vi "Text control 2 v3.9.vi"() -> ()   [LabVIEW 2016]
panel:
  in  "Tab Control":enum32{"Main", "Other parameters"}(tab)
  out "Line running":i32
  out "Total lines":i32
  out "Path":path=path "C:/users/rlp38/09Apr2009LTtesting/test2.txt"
  out "I vs Vg":cluster{"Y data in":dbl[], "X data in":dbl[]}[](graph)
  out "Is":dbl format="%.2e"
  out "Id":dbl format="%.2e"
  out "Ig":dbl format="%.2e"
  out "Id max vs time":cluster{"Y data in":dbl[], "X data in":dbl[]}[](graph)
  out "Id min vs time":cluster{"Y data in":dbl[], "X data in":dbl[]}[](graph)
  out "I vs Vd":cluster{"Y data in":dbl[], "X data in":dbl[]}[](graph)
  in  "Program":string="#pulsedstressV d 0.03 20 0 0.5 0.0827 5\n#\n#itime s\n#gaterangemode l\n#drainrangemode l\n#serial /1Q #query pump\n#wait 1000 #wait 1 second\n#serial /1ZR #initialize pump\n#wait 20000 #wait 20 seconds\n#serial /1V300R #choose speed: 300 steps/s\n#wait 1000 #wait 1 second\n#serial /1O3R #go to port 3, counterclockwise rotation\n#wait 1000 #wait 1 second\n#serial /1A2400R #go to absolute position 2400\n#wait 1000 #wait 1 second\n#serial /1? #report absolute plunger position\n#serial /1V80R #set speed to 80 steps/s\n#serial /1O5 #switch to port 5, counterclockwise rotation\n#wait 200 #wait 200 milliseconds\n#serial /1A0R #go to absolute position 0 (= empty syringe)\n#serial /1? #report absolute plunger position\n#pulsed on 0.05 0 0.02\n#transfer d 1 -1 -0.1 -1 -1 0\n#wait-min 1\n#transfer d 1 -1 -0.1 -1 -1 0\n#output d 0 -1 -0.5 0 -1 -0.1\n#transfer d -10 40 1 5 40 35\n#transfer d -10 40 1 5 40 35\n#output d 0 40 20 0 40 1\n#\n#\n#sample 1 0.008 221 6 0.003\n#samplei 400e-6 200 6 0.002 0.1\n#vsu2pulse -10 4\n#\n#stressV 0.016 0.03 2e-4 0.1e-3 11\n#stressI 220e-7 0.08 15\n#transfer s -1 1 0.5 -0.005 0.005 0.005\n#output s 0 0 0 -0.008 0.008 0.002"
  out "Command running:":string="#output s 0 0 0 -0.008 0.008 0.002"
  out "Serial port output":string
  in  "Step delay /s":dbl format="%.2f"
  in  "Integration time (long)":dbl=0.32 min=0.04 max=2.0 step=0.02 format="%.2f"
  in  "Integration time (short)":dbl=0.0019 min=8e-05 max=0.0019 step=8e-05 format="%^.0e"
  in  "integration time":u32(slide) max=2 step=1 scale=0.0..2.0
  in  "delay time /s":dbl format="%.2f"
  in  "hold time /s":dbl format="%.2f"
  in  "Gate: Compliance":dbl=0.001 format="%.8f"
  in  "Drain: Compliance":dbl=0.001 format="%.8f"
  in  "Interrupt run":bool
  out "Elapsed Time":dbl caption="Elapsed Time (s)"
  in  "Units":u16(ring) items=["Seconds", "Minutes", "Hours"]
  in  "Time Offset":dbl caption="Set Start Time (s)"
  in  "Reset":bool
  in  "Auto Reset":bool
  in  "Gate Range\nmode":u16(ring) items=["Auto", "Limited", "Fixed"]
  in  "Gate Range":u8(slide)=6 max=11 scale=0.0..11.0
  in  "Source/Drain\nRange mode":u16(ring) items=["Auto", "Limited", "Fixed"]
  in  "Source/Drain Range":u8(slide)=6 max=11 scale=0.0..11.0
  in  "Panel Controls":T1={"Emergency Stop"=refnum, "TransGraph Max"=1e-05, "Text/Graph (text=false)"=TRUE} {"TransGraph Max" format="%.2e"}
  in  "Panel Controls 2":T2={"Emergency Stop"=refnum, "TransGraph Max"=1e-05, "Text/Graph (text=false)"=TRUE, "TransGraph Min"=1e-11} {"TransGraph Min" format="%.2e"; "TransGraph Max" format="%.2e"}
  in  "SMU4":cluster{"on/off":bool, "Voltage":dbl} {"Voltage" min=-100.0 max=100.0 format="%.2f"}
  in  "Full Reset":bool
  in  "Standby":T3
  in  "Delay before read (ms)":u32=1000
  in  "byte count":u32=64
  in  "Serial End Mode for Reads":u16(ring)=2 items=["None", "LastBit", "TermChar"]
  in  "Timeout (ms)":u32=10000
  in  "Enable Termination\nChar (T)":bool=TRUE
  in  "Termination char\n(0xA = '\\n' = LF)\n(0xD = '\\r' = CR)":u8=13 format="%.0x"
  in  "flow control":u16(ring) items=["None"=0, "XON/XOFF"=1, "RTS/CTS"=2, "DTR/DSR"=4]
  in  "stop bits":u16(ring)=10 items=["1.0"=10, "1.5"=15, "2.0"=20]
  in  "parity":u16(ring) items=["None", "Odd", "Even", "Mark", "Space"]
  in  "data bits":u16=8 min=5 max=8 step=1
  in  "VISA resource name":refnum<visa-resource-name>="COM6"
  in  "baud rate":u32=9600
  out "error out":errorcluster
  in  "Gate":T4={"Gate Start"=0.0, "Gate Stop"=2.0, "Gate Step (linear only)"=1.0, "Gate Compliance"=0.0001, "Gate PComp"=0.0, "Range mode"=0, "Range"=6} {"Range" max=11 scale=0.0..11.0; "Range mode" items=["Auto", "Limited", "Fixed"]; "Gate PComp" format="%^.2e"; "Gate Compliance" format="%^.2e"; "Gate Step (linear only)" format="%^.4e"; "Gate Stop" format="%^.4e"; "Gate Start" format="%^.4e"}
  in  "Drain 2":T5={"Drain Start"=0.0, "Drain Stop"=2.0, "Drain Compliance"=0.0001, "Drain Step"=1.0, "Drain PComp"=0.0, "Range mode"=0, "Range"=6} {"Range" max=11 scale=0.0..11.0; "Range mode" items=["Auto", "Limited", "Fixed"]; "Drain PComp" format="%^.2e"; "Drain Step" format="%^.4e"; "Drain Compliance" format="%^.2e"; "Drain Stop" format="%^.4e"; "Drain Start" format="%^.4e"}
  in  "Timings 2":T6={"integration time"=0, "Short/Long integration time"=0.00064, "hold time (sec)"=0.0, "delay time (sec)"=0.0, "Step Time (0 disables)"=0.0, "sweep method"=0, "Pulse period"=0.005, "Base voltage"=0.0, "Pulse width"=0.0005} {"Pulse width" min=0.0005 max=0.1 step=0.0001 format="%.4f"; "Base voltage" format="%^.4e"; "Pulse period" min=0.005 max=1.0 step=0.0001 format="%.4f"; "sweep method" items=["Continuous", "Pulsed"]; "Step Time (0 disables)" format="%.2f"; "delay time (sec)" format="%.4f"; "hold time (sec)" format="%.4f"; "Short/Long integration time" format="%^.0e"; "integration time" scale=0.0..2.0}
  # "Time"
  # "1\n2\n3\n4\n5\n6\n7\n8\n9\n10\n11\n12\n13\n14\n15\n16\n17\n18\n19\n20\n21\n22\n23\n24\n25"
  # "Syntax:\nitime [s|m|l]\ngaterangemode [a|l|f]\ndrainrangemode [a|l|f]\npulsed [on|off] PulsePeriod(sec) PulseBaseVoltage PulseONWidth(sec)\nstandby [on l off]\nwait NumMilliseconds\nwait-min NumMinutes\n# texthere = comment\ntransfer [s|d] VgStart VgStop VgStep VdStart VdStop VdStep\noutput [s|d] VgStart VgStop VgStep VdStart VdStop VdStep\nsample Vg Vd NumSamples Time(s) SampleInterval(s)\nsamplei Idg NumSamples Time(s) SampleInterval(s) VDGcompliance\n100 samples is approximately 13 seconds with medium integration\n# if in doubt use SampleInterval(s) = 0.004\nstressV VG VD IGcompliance IDcompliance Duration(sec)\nstressI IDG VDGcompliance Duration(sec)\nvsu2pulse Bias Duration(s)\npulsedstressV [s|d] VEstop VgON VgOFF Period(s) PulseONwidth(s) Vd\nsample-fpp Vg Vd NumSamples Time\nresample-fpp Vg Vd\ntransfer-fpp [s|d] VgStart VgStop VgStep VdStart VdStop VdStep\noutput-fpp [s|d] VgStart VgStop VgStep VdStart VdStop VdStep\nserial SerialPortCommand"
  # "Serial port settings"
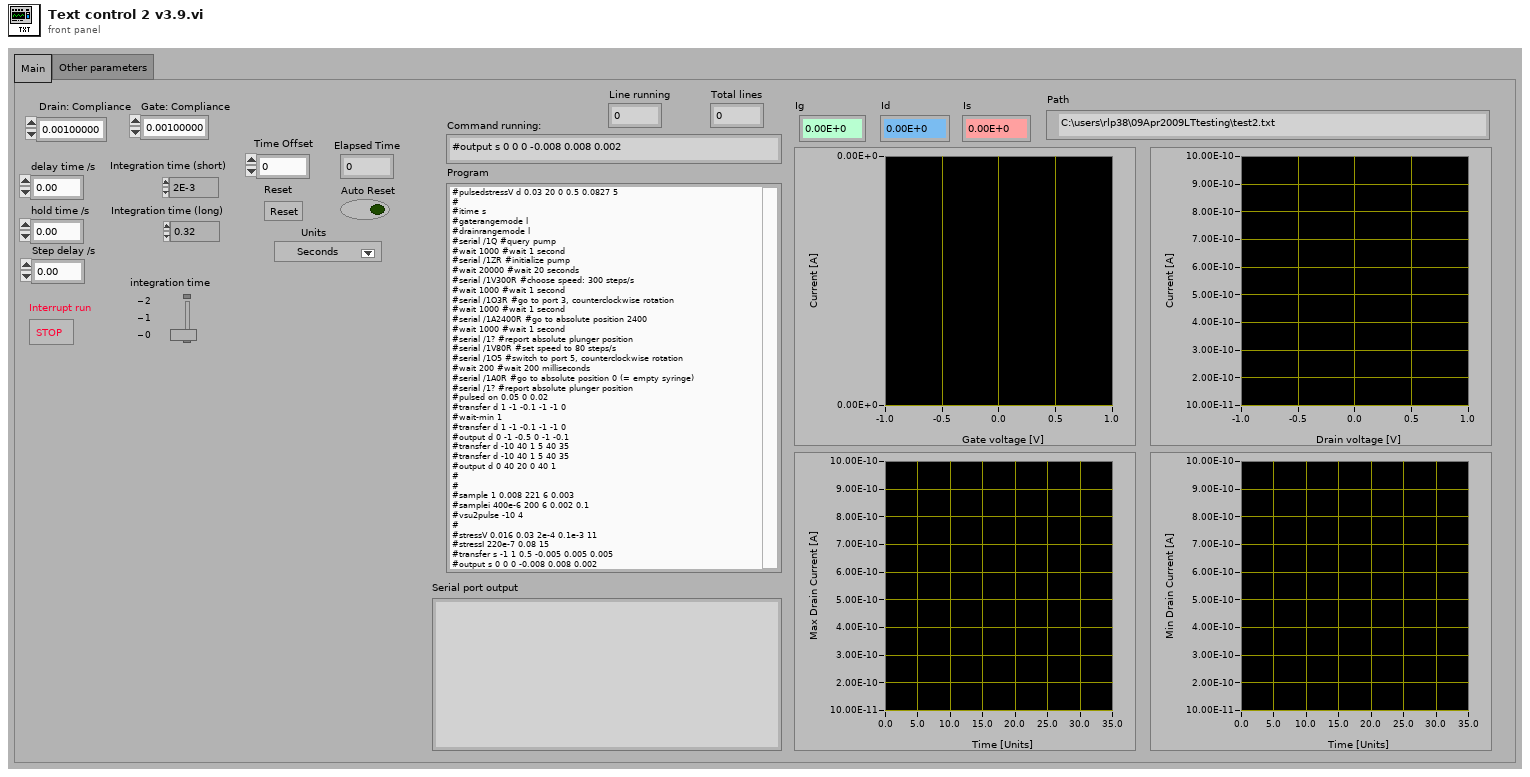
[diagram p1: front panel]
types:
  T1 = cluster{"Emergency Stop":refnum<vi>, "TransGraph Max":dbl, "Text/Graph (text=false)":bool}
  T2 = cluster{"Emergency Stop":refnum<vi>, "TransGraph Max":dbl, "Text/Graph (text=false)":bool, "TransGraph Min":dbl}
  T3 = cluster{"Gate Standby":bool, "Drain Standby":bool}
  T4 = cluster{"Gate Start":dbl, "Gate Stop":dbl, "Gate Step (linear only)":dbl, "Gate Compliance":dbl, "Gate PComp":dbl, "Range mode":u16, "Range":u8}
  T5 = cluster{"Drain Start":dbl, "Drain Stop":dbl, "Drain Compliance":dbl, "Drain Step":dbl, "Drain PComp":dbl, "Range mode":u16, "Range":u8}
  T6 = cluster{"integration time":u32, "Short/Long integration time":dbl, "hold time (sec)":dbl, "delay time (sec)":dbl, "Step Time (0 disables)":dbl, "sweep method":u16, "Pulse period":dbl, "Base voltage":dbl, "Pulse width":dbl}
  T7 = enum16{"open", "replace", "create", "open or create", "replace or create", "replace or create with confirmation"}
  T8 = cluster{"V2 Start":dbl, "V2 Step":dbl, "Number of points":i32}
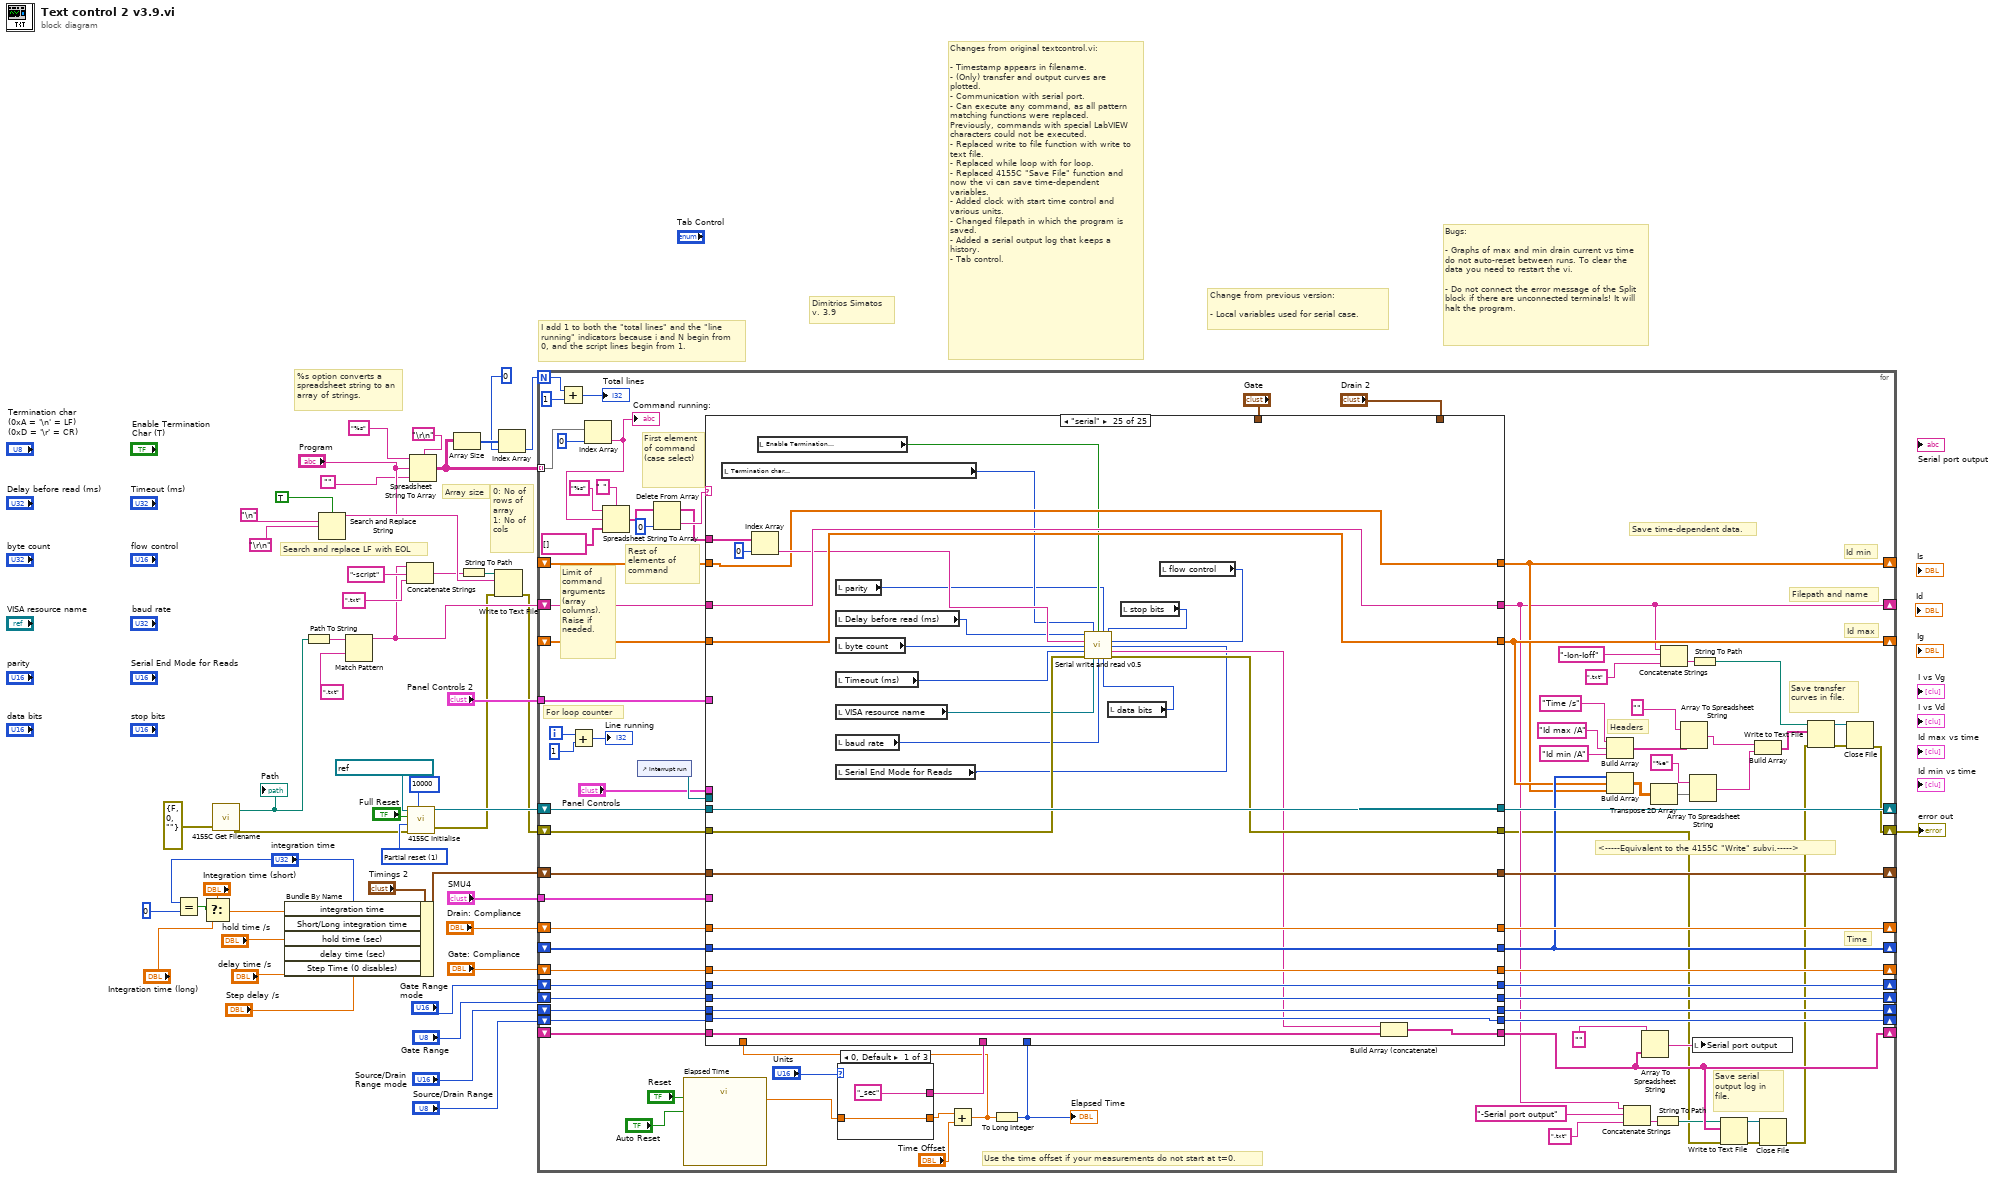
[diagram p0: block diagram]
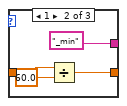
[diagram p2: hidden frame]
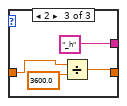
[diagram p3: hidden frame]
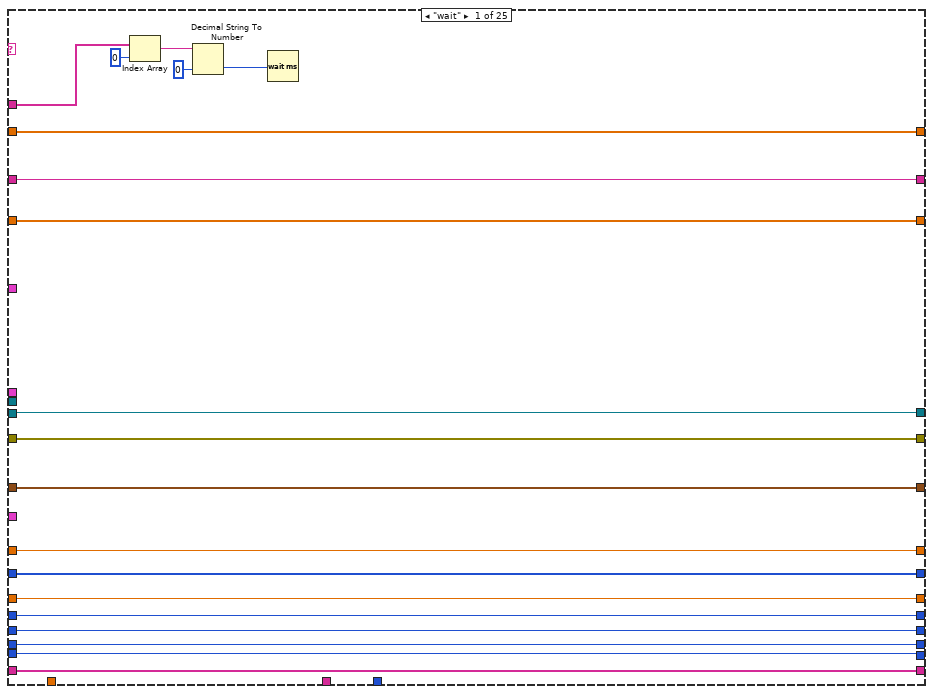
[diagram p4: hidden frame]
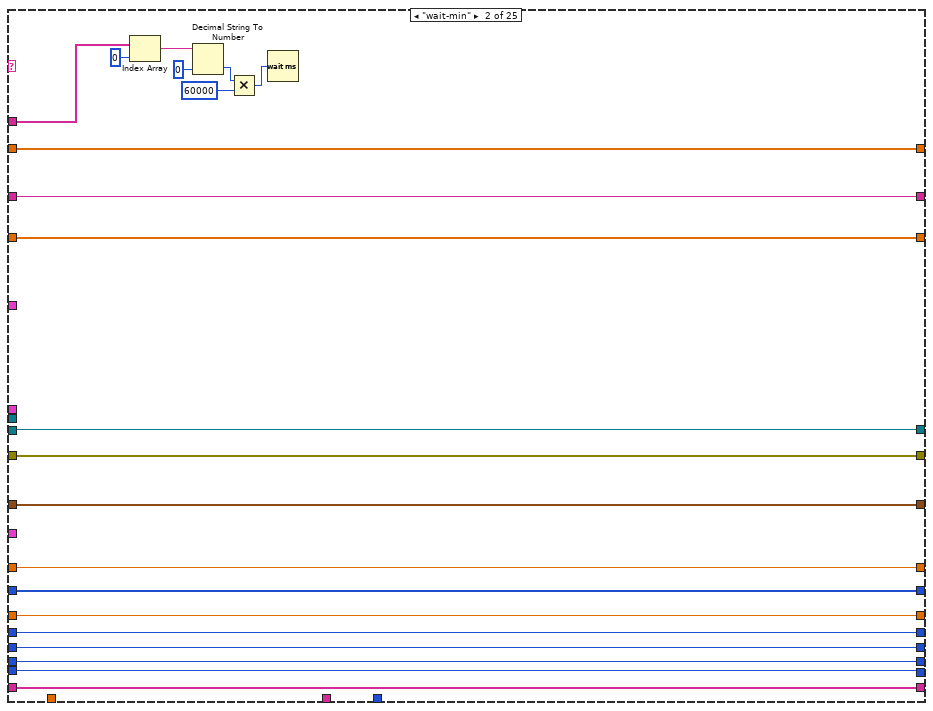
[diagram p5: hidden frame]
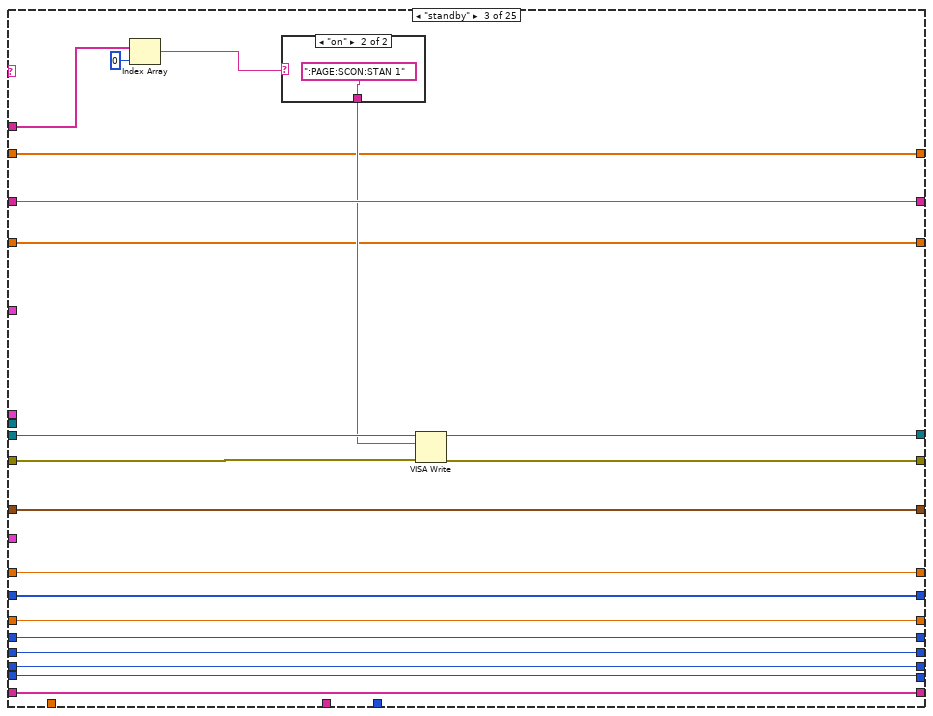
[diagram p6: hidden frame]
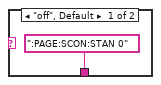
[diagram p7: hidden frame]
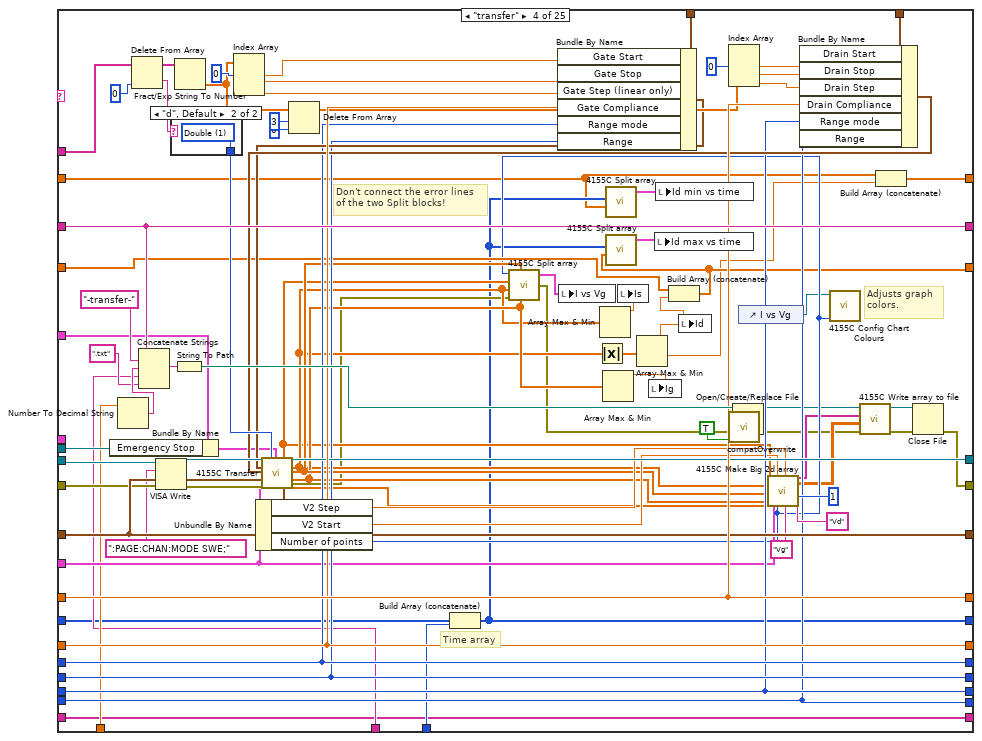
[diagram p8: hidden frame]
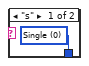
[diagram p9: hidden frame]
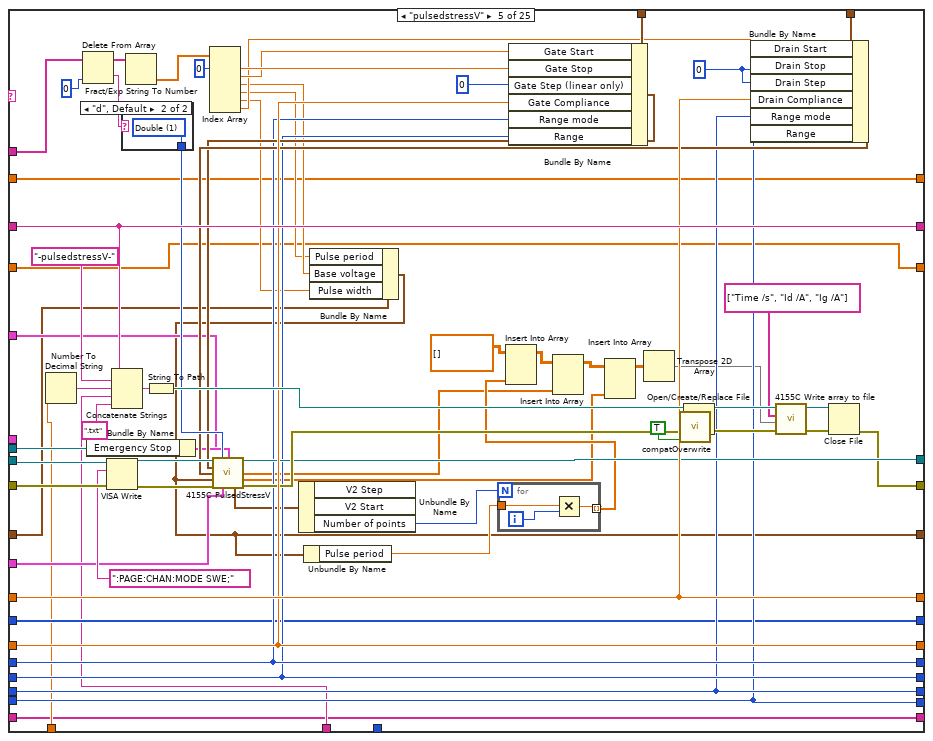
[diagram p10: hidden frame]
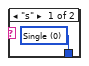
[diagram p11: hidden frame]
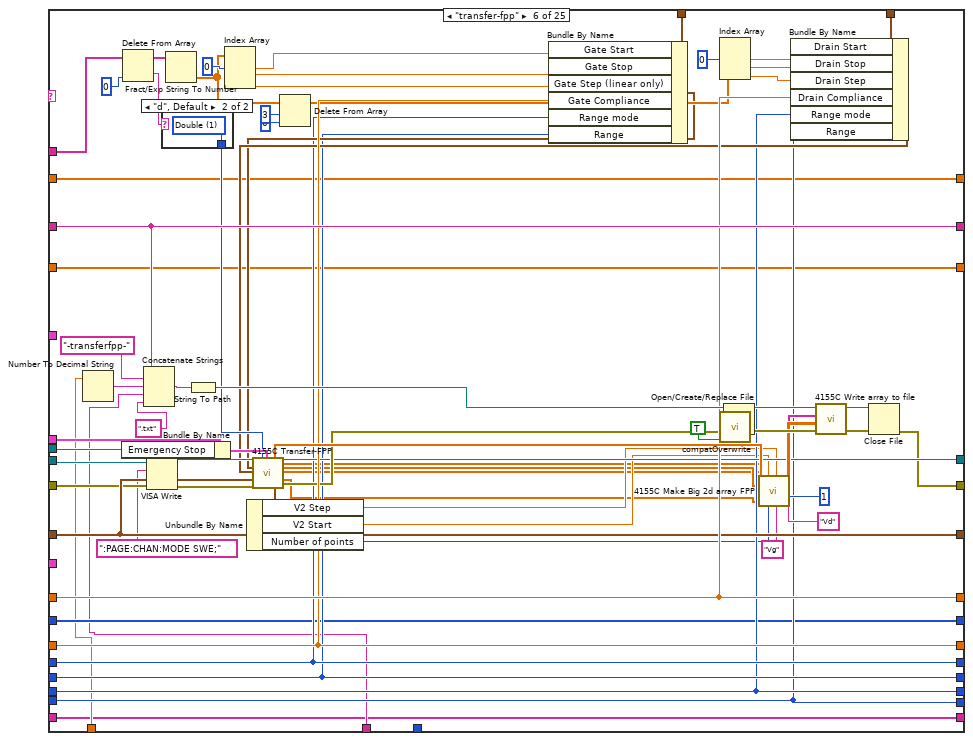
[diagram p12: hidden frame]
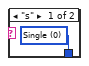
[diagram p13: hidden frame]
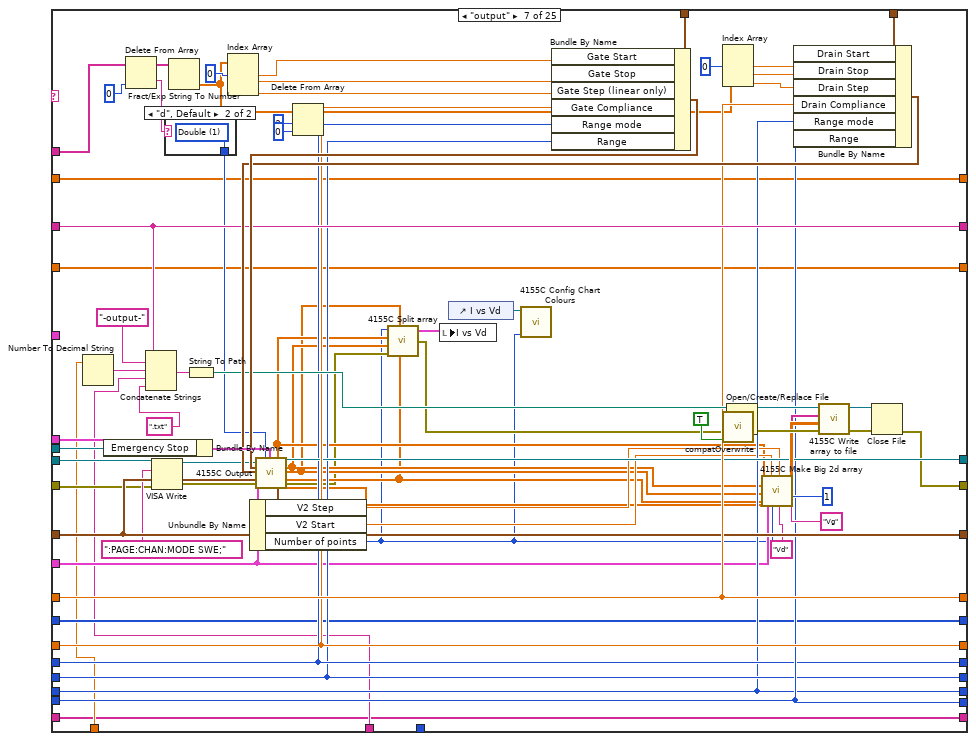
[diagram p14: hidden frame]
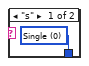
[diagram p15: hidden frame]
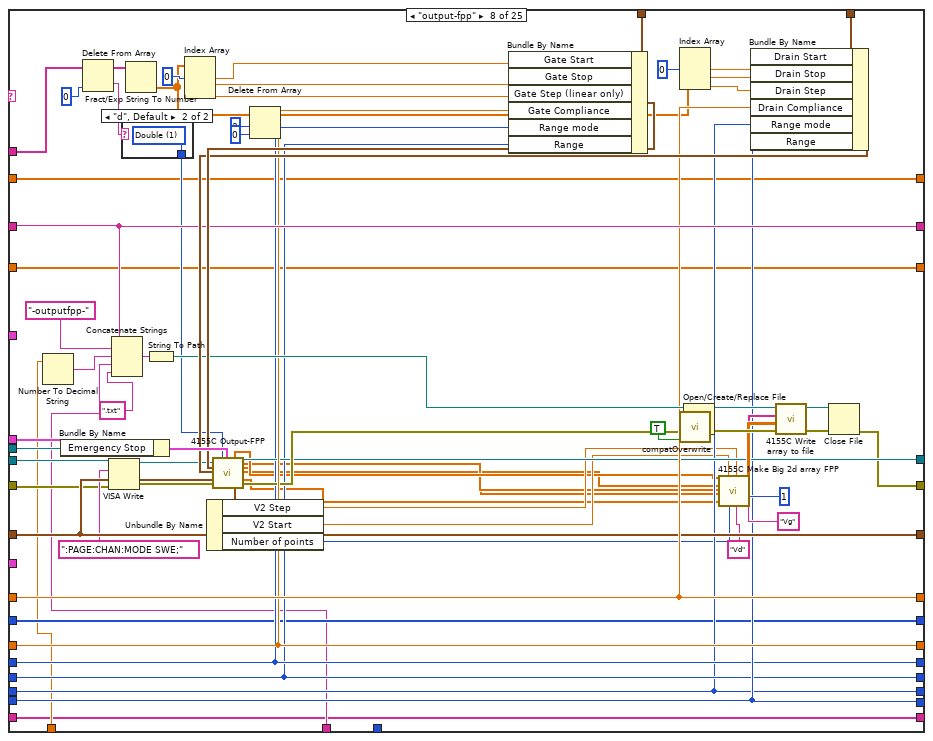
[diagram p16: hidden frame]
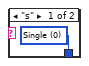
[diagram p17: hidden frame]
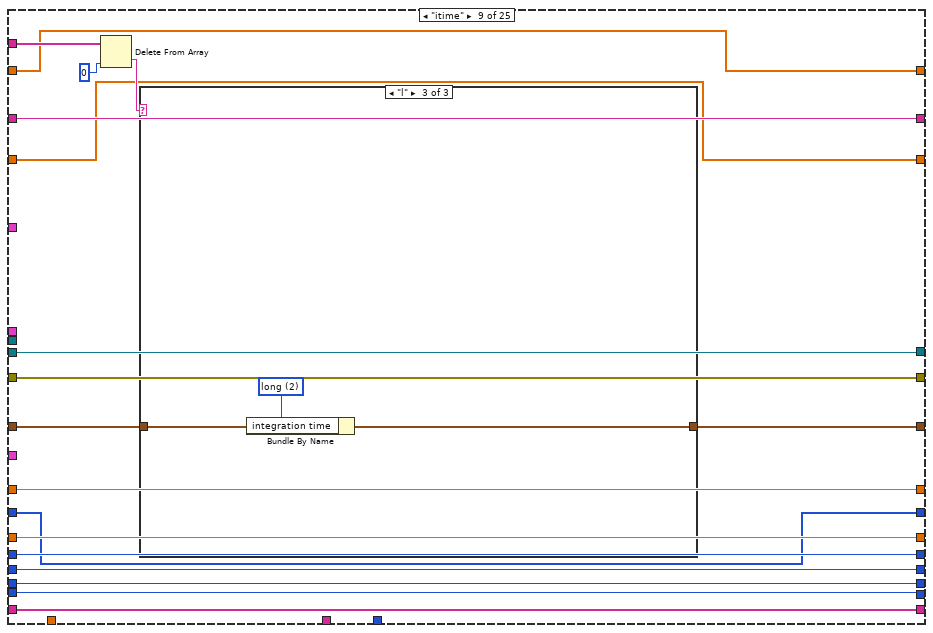
[diagram p18: hidden frame]
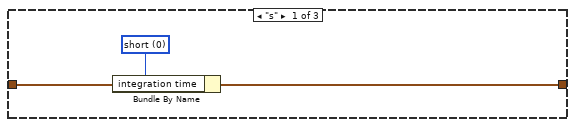
[diagram p19: hidden frame]
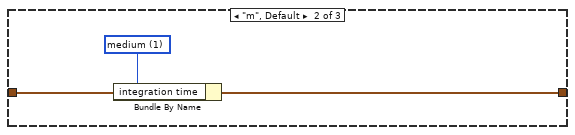
[diagram p20: hidden frame]
diagram:
  w40 = u16 1 items=["Reset All", "Partial reset"] ("Type of reset")
  # "Change from previous version:\n\n- Local variables used for serial case."
  # "I add 1 to both the \"total lines\" and the \"line running\" indicators because i and N begin from 0, and the script lines begin from 1."
  # "Bugs:\n\n- Graphs of max and min drain current vs time do not auto-reset between runs. To clear the data you need to restart the vi.\n\n- Do not connect the error message of the Split block if there are unconnected terminals! It will halt the program."
  # "Array size"
  # "%s option converts a spreadsheet string to an array of strings."
  # "0: No of rows of array\n1: No of cols"
  # "Dimitrios Simatos\nv. 3.9"
  # "Changes from original textcontrol.vi:\n\n- Timestamp appears in filename.\n- (Only) transfer and output curves are plotted.\n- Communication with serial port.\n- Can execute any command, as all pattern matching functions were replaced. Previously, commands with special LabVIEW characters could not be executed.\n- Replaced write to file function with write to text file.\n- Replaced while loop with for loop.\n- Replaced 4155C \"Save File\" function and now the vi can save time-dependent variables.\n- Added clock with start time control and various units.\n- Changed filepath in which the program is saved.\n- Added a serial output log that keeps a history.\n- Tab control."
  # "Search and replace LF with EOL"
  n1 = Equal?(x="integration time", y=u32 0) -> (x = y?=w44:bool)
  n2 = Select(t="Integration time (short)", s=w44, f="Integration time (long)") -> (s? t:f=w48:dbl)
  n3 = call "4155C Get Filename.vi"("error in (no error)"=errorcluster {"status"=FALSE, "code"=0, "source"=""}) -> ("error out"=w35:errorcluster, "path"=w10:path)  [unwired: 2 in, 1 out]
  "Path" <- w10
  n4 = Bundle By Name(cluster="Timings 2", "integration time"="integration time", "Short/Long integration time"=w48, "hold time (sec)"="hold time /s", "delay time (sec)"="delay time /s", "Step Time (0 disables)"="Step delay /s") -> (w33:T6)
  n5 = Path To String(path=w10) -> (string=w11:string)
  n6 = Search and Replace String(replace all?=TRUE ("replace all? (F)"), input string="Program", search string="\n", replace string="\r\n") -> (result string=w23:string)  [unwired: 4 in, 3 out]
  n7 = Match Pattern(string=w11, regular expression=".txt") -> (before substring=w5:string)  [unwired: 1 in, 3 out]
  n8 = Concatenate Strings(w5, "-script" ("Prefix"), ".txt" ("regular expression")) -> (w4:string)
  n9 = call "4155C Initialise.vi"("VISA resource name in"=refnum<visa-resource-name> "GPIB0::14::INSTR", "Reset"="Full Reset", "Type of reset"=w40, "error in (no error)"=w35, "VISA Timeout Value"=u32 10000) -> ("VISA Resource Name out"=w34:refnum<visa-resource-name>, "error out"=w2:errorcluster)
  n10 = Spreadsheet String To Array(delimiter (Tab)="\r\n", format string="%s", spreadsheet string="Program", array type (2D Dbl)="") -> (array=w14:string[][])
  n11 = Array Size(array=w14) -> (size(s)=w18:i32[])
  n12 = String To Path(string=w4) -> (path=w3:path)
  n13 = Write to Text File(file (use dialog)=w3, text=w23, error in=w2) -> (error out=w1:errorcluster)  [unwired: 1 in, 2 out]
  n14 = Index Array(array=w18, index=0) -> (element=w16:i32)
  n15 = for {
    N: w16 -> [w68]
    tunnel: "SMU4" -> [w113]
    shift-left: "Source/Drain Range" -> [w118]
    shift-right: [w114] -> _
    shift-left: "Source/Drain\nRange mode" -> [w119]
    shift-right: [w115] -> _
    shift-left: "Gate Range" -> [w120]
    shift-right: [w116] -> _
    shift-left: "Gate Range\nmode" -> [w121]
    shift-right: [w117] -> _
    shift-left: "Gate: Compliance" -> [w130]
    shift-right: [w126] -> _
    shift-left: "Drain: Compliance" -> [w131]
    shift-right: [w127] -> _
    shift-left: w33 -> [w132]
    shift-right: [w128] -> _
    shift-left: w1 -> [w133]
    shift-right: [w76] -> w9
    shift-left: w34 -> [w134]
    shift-right: [w129] -> _
    shift-left: w5 -> [w135]
    shift-right: [w52] -> _
    tunnel: "Panel Controls 2" -> [w112]
    shift-right: [w80] -> _
    shift-left: _ -> [w111]
    shift-right: [w81] -> _
    shift-left: _ -> [w107]
    tunnel: w14 -> [w105] mode=indexing
    shift-right: [w74] -> _
    shift-left: _ -> [w75]
    shift-right: [w57] -> _
    shift-left: _ -> [w60]
    i -> [w63]
    # "Save serial output log in file."
    # "For loop counter"
    # "<-----Equivalent to the 4155C \"Write\" subvi.----->"
    # "Headers"
    # "Save transfer curves in file."
    # "Filepath and name"
    # "Save time-dependent data."
    # "Use the time offset if your measurements do not start at t=0."
    # "Time"
    # "Rest of elements of command"
    # "Id min"
    # "Id max"
    # "Limit of command arguments (array columns). Raise if needed."
    # "First element of command\n(case select)"
    n16 = Add(x=w68, y=1) -> (x+y=→"Total lines":i32)
    n17 = Add(x=w63, y=1) -> (x+y=→"Line running":i32)
    n18 = Index Array(array=w105, index=0 ("line index")) -> (element=w100:string)
    "Command running:" <- w100
    n19 = Spreadsheet String To Array(delimiter (Tab)=" ", format string="%s", spreadsheet string=w100, array type (2D Dbl)=string[] []) -> (array=w97:string[])
    n20 = control-ref of="Interrupt run"() -> (w125:refnum<vi>)
    n21 = Delete From Array(array=w97, index=0) -> (deleted portion=w98:string, array with subset deleted=w96:string[])  [unwired: 1 in]
    n22 = call "Elapsed Time"("Reset"="Reset", "Auto Reset"="Auto Reset") -> ("Elapsed Time (s)"=w108:dbl)  [unwired: 10 in, 7 out]
    n23 = case shown="0, Default" "Units" {
      tunnel: ["_sec" "_min" "_h"] -> w109
      tunnel: [w136 w140 w143] -> w70
      tunnel: w108 -> [w136 w139 w144]
      frame 0, Default {
      }
      frame 1 {
        n24 = Divide(x=w139, y=60.0) -> (x/y=w140:dbl)
      }
      frame 2 {
        n25 = Divide(x=w144, y=3600.0) -> (x/y=w143:dbl)
      }
    }
    n26 = Add(x=w70, y="Time Offset") -> (x+y=w69:dbl)
    n27 = To Long Integer(number=w69) -> (32bit integer=w106:i32)
    "Elapsed Time" <- w106
    n28 = case shown="\"serial\"" w98 {
      tunnel: w96 -> [w164 w185 w205 w282 w348 w419 w496 w568 w608 w636 w665 w692 w715 w731 _ _ w841 w904 _ w973 w1019 w1063 w1135 w1199 w1221]
      tunnel: w135 -> [w159 w181 w203 w289 w355 w427 w503 w576 w597 w625 w657 w685 w709 w724 w745 w789 w819 w886 w919 w960 w1006 w1051 w1129 w1195 w1223]
      tunnel: w134 -> [w158 w180 w194 w260 w339 w396 w472 w544 w598 w626 w658 w686 w710 w725 w750 w791 w847 w910 w923 w979 w1025 w1069 w1141 w1153 w1227]
      tunnel: w133 -> [w157 w179 w193 w259 w338 w395 w469 w541 w599 w627 w659 w687 w711 w726 w749 w762 w846 w909 w922 w978 w1024 w1068 w1140 w1152 w1226]
      tunnel: w132 -> [w156 w178 w202 w285 w314 w423 w499 w572 w607 w635 w656 w684 w708 w723 w748 w786 w810 w878 w928 w953 w999 w1044 w1128 w1194 w1228]
      tunnel: w131 -> [w155 w177 w201 w287 w353 w425 w501 w574 w606 w634 w664 w691 w714 w730 w747 w771 w845 w908 w931 w977 w1023 w1067 w1139 w1203 w1229]
      tunnel: w130 -> [w154 w176 w200 w286 w352 w424 w500 w573 w605 w633 w663 w690 w713 w729 w746 w772 w820 w887 w930 w961 w1007 w1052 w1130 w1196 w1231]
      tunnel: [w158 w180 w192 w284 w350 w421 w498 w570 w598 w626 w658 w686 w710 w725 w750 w791 w811 w860 w921 w954 w1000 w1045 w1081 w1155 w1227] -> w129
      tunnel: [w157 w179 w191 w283 w349 w420 w497 w569 w599 w627 w659 w687 w711 w726 w749 w761 w821 w861 w920 w962 w1008 w1053 w1080 w1154 w1225] -> w51
      tunnel: [w156 w178 w202 w285 w310 w423 w499 w572 w600 w628 w656 w684 w708 w723 w748 w786 w810 w878 w928 w953 w999 w1044 w1128 w1194 w1228] -> w128
      tunnel: [w155 w177 w201 w287 w353 w425 w501 w574 w606 w634 w664 w691 w714 w730 w747 w771 w845 w908 w931 w977 w1023 w1067 w1139 w1203 w1229] -> w127
      tunnel: [w154 w176 w200 w286 w352 w424 w500 w573 w605 w633 w663 w690 w713 w729 w746 w772 w820 w887 w930 w961 w1007 w1052 w1130 w1196 w1231] -> w126
      tunnel: [w159 w181 w203 w289 w355 w427 w503 w576 w597 w625 w657 w685 w709 w724 w745 w789 w819 w886 w919 w960 w1006 w1051 w1129 w1195 w1223] -> w52
      tunnel: w125 -> [_ _ _ w292 w359 w432 w507 w580 _ _ _ _ _ _ _ _ w816 w883 _ w959 w1005 w1050 w1101 w1171 _]
      tunnel: "Gate" -> [_ _ _ w269 w342 w406 w483 w555 _ _ _ _ _ _ _ _ _ _ _ _ _ _ _ _ _]
      tunnel: "Drain 2" -> [_ _ _ w268 w341 w405 w482 w554 _ _ _ _ _ _ _ _ _ _ _ _ _ _ _ _ _]
      tunnel: "Panel Controls" -> [_ _ _ _ _ w404 w481 w553 _ _ _ _ _ _ _ _ _ _ _ _ _ _ _ _ _]
      tunnel: w121 -> [w153 w175 w199 w253 w332 w389 w467 w539 w604 w632 _ w683 w707 w722 w744 w773 w806 w874 w924 w949 w995 w1040 w1124 w1190 w1232]
      tunnel: w120 -> [w152 w174 w198 w252 w331 w388 w466 w538 w603 w631 w662 _ w698 w728 w743 w774 w807 w875 w925 w950 w996 w1041 w1125 w1191 w1233]
      tunnel: w119 -> [w151 w173 w197 w251 w330 w387 w465 w537 w602 w630 w661 w689 w712 _ w742 w775 w808 w876 w926 w951 w997 w1042 w1126 w1192 w1234]
      tunnel: w118 -> [w150 w172 w196 w250 w329 w386 w468 w540 w601 w629 w660 w688 _ w727 w741 w776 w809 w877 w927 w952 w998 w1043 w1127 w1193 w1235]
      tunnel: [w153 w175 w199 w253 w332 w389 w467 w539 w604 w632 w655 w683 w707 w722 w744 w773 w806 w874 w924 w949 w995 w1040 w1124 w1190 w1232] -> w117
      tunnel: [w152 w174 w198 w252 w331 w388 w466 w538 w603 w631 w662 w675 w698 w728 w743 w774 w807 w875 w925 w950 w996 w1041 w1125 w1191 w1233] -> w116
      tunnel: [w151 w173 w197 w251 w330 w387 w465 w537 w602 w630 w661 w689 w712 w721 w742 w775 w808 w876 w926 w951 w997 w1042 w1126 w1192 w1234] -> w115
      tunnel: [w150 w172 w196 w250 w329 w386 w468 w540 w601 w629 w660 w688 w699 w727 w741 w776 w809 w877 w927 w952 w998 w1043 w1127 w1193 w1235] -> w114
      tunnel: w113 -> [_ _ _ w245 w326 _ w461 _ _ _ _ _ _ _ _ _ _ _ _ _ _ _ _ _ _]
      tunnel: w112 -> [_ _ _ w243 w325 _ _ _ _ _ _ _ _ _ _ _ _ _ _ _ _ _ _ _ _]
      tunnel: [w149 w168 w189 w220 w302 w376 w458 w526 w596 w623 w654 w674 w697 w720 w740 w757 w798 w858 w918 w938 w988 w1034 w1078 w1148 w1224] -> w80
      tunnel: w111 -> [w149 w168 w189 w234 w302 w376 w458 w526 w596 w623 w654 w674 w697 w720 w740 w757 w798 w858 w918 w938 w988 w1034 w1078 w1148 w1224]
      tunnel: w69 -> [_ _ _ w230 w299 w374 w455 w523 _ _ _ _ _ _ _ w755 w796 w855 _ w935 w985 w1031 w1075 w1144 _]
      tunnel: w109 -> [_ _ _ w227 w298 w372 w454 w522 _ _ _ _ _ _ _ w753 w794 w854 _ w934 w984 w1030 w1074 w1145 _]
      tunnel: w106 -> [_ _ _ w221 _ _ _ _ _ _ _ _ _ _ _ _ _ _ _ _ _ _ _ _ _]
      tunnel: [w148 w167 w188 w218 w301 w375 w457 w525 w595 w622 w653 w673 w696 w719 w739 w756 w797 w857 w917 w937 w987 w1033 w1077 w1147 w1230] -> w81
      tunnel: w107 -> [w148 w167 w188 w226 w301 w375 w457 w525 w595 w622 w653 w673 w696 w719 w739 w756 w797 w857 w917 w937 w987 w1033 w1077 w1147 w1230]
      tunnel: [w147 w166 w187 w216 w297 w371 w453 w521 w594 w621 w652 w672 w695 w718 w738 w752 w793 w853 w916 w933 w983 w1029 w1073 w1143 w1219] -> w74
      tunnel: w75 -> [w147 w166 w187 w215 w297 w371 w453 w521 w594 w621 w652 w672 w695 w718 w738 w752 w793 w853 w916 w933 w983 w1029 w1073 w1143 w1219]
      tunnel: [w146 w165 w186 w208 w296 w370 w443 w520 w593 w620 w651 w671 w694 w717 w737 w751 w792 w852 w915 w932 w982 w1028 w1072 w1142 w1217] -> w57
      tunnel: w60 -> [w146 w165 w186 w208 w296 w370 w443 w520 w593 w620 w651 w671 w694 w717 w737 w751 w792 w852 w915 w932 w982 w1028 w1072 w1142 w1216]
      frame "wait" {
        n29 = Index Array(array=w164, index=0 ("Index")) -> (element=w162:string)
        n30 = Decimal String To Number(string=w162, default (0L)=u32 0) -> (number=w161:u32)  [unwired: 1 in, 1 out]
        n31 = Wait (ms)(milliseconds to wait=w161) -> ()  [unwired: 1 out]
      }
      frame "wait-min" {
        n32 = Index Array(array=w185, index=0 ("Index")) -> (element=w183:string)
        n33 = Decimal String To Number(string=w183, default (0L)=u32 0) -> (number=w171:u32)  [unwired: 1 in, 1 out]
        n34 = Multiply(x=w171, y=u32 60000) -> (x*y=w170:u32)
        n35 = Wait (ms)(milliseconds to wait=w170) -> ()  [unwired: 1 out]
      }
      frame "standby" {
        n36 = Index Array(array=w205, index=0 ("Index")) -> (element=w195:string)
        n37 = case shown="\"on\"" w195 {
          tunnel: [":PAGE:SCON:STAN 0" ":PAGE:SCON:STAN 1"] -> w190
          frame "off", Default {
          }
          frame "on" {
          }
        }
        n38 = VISA Write(VISA resource name=w194, write buffer=w190, error in (no error)=w193) -> (VISA resource name out=w192:refnum<visa-resource-name>, error out=w191:errorcluster)  [unwired: 1 out]
      }
      frame "transfer" {
        # "Don't connect the error lines\nof the two Split blocks!"
        # "Adjusts graph colors."
        # "Time array"
        n39 = Bundle By Name(cluster=w243, "Emergency Stop"=w292) -> (w244:T2)
        n40 = Number To Decimal String(number=w230) -> (decimal integer string=w229:string)  [unwired: 1 in]
        n41 = Delete From Array(array=w282, index=0 ("Index")) -> (deleted portion=w280:string, array with subset deleted=w279:string[])  [unwired: 1 in]
        n42 = Concatenate Strings(w289, "-transfer-" ("Prefix"), w229, w227, ".txt" ("Suffix")) -> (w291:string)
        n43 = VISA Write(VISA resource name=w260, write buffer=":PAGE:CHAN:MODE SWE;" ("write buffer (\"\")"), error in (no error)=w259) -> (VISA resource name out=w257:refnum<visa-resource-name>, error out=w258:errorcluster)  [unwired: 1 out]
        n44 = case shown="\"d\", Default" w280 {
          tunnel: [w294 w295] -> w278
          frame "s" {
            w294 = u16 0 items=["Single", "Double"] ("sweep mode")
          }
          frame "d", Default {
            w295 = u16 1 items=["Single", "Double"] ("sweep mode")
          }
        }
        n45 = String To Path(string=w291) -> (path=w288:path)
        n46 = Fract/Exp String To Number(string=w279) -> (number=w264:dbl[])  [unwired: 3 in, 1 out]
        n47 = Index Array(array=w264, index #1=0 ("Index")) -> (element #1=w277:dbl, element #2=w276:dbl, element #3=w275:dbl)  [unwired: 2 in]
        n48 = Delete From Array(array=w264, length=3 ("Length"), index=0 ("Index")) -> (array with subset deleted=w262:dbl[])  [unwired: 1 out]
        n49 = Build Array (concatenate)(w226, w221) -> (w218:i32[])
        n50 = Bundle By Name(cluster=w269, "Gate Start"=w277, "Gate Stop"=w276, "Gate Step (linear only)"=w275, "Gate Compliance"=w286, "Range mode"=w253, "Range"=w252) -> (w254:T4)
        n51 = call "4155C Split array.vi"("X data in"=w218, "Y1 data in"=w215) -> ("Array of clusters"=w219:cluster{"Y data in":dbl[], "X data in":dbl[]}[])  [unwired: 5 in, 1 out]
        n52 = local write "Id min vs time"(w219) -> ()
        n53 = Index Array(array=w262, index #1=0 ("Index")) -> (element #1=w272:dbl, element #2=w271:dbl, element #3=w270:dbl)  [unwired: 2 in]
        n54 = call <vilib>:"compatOverwrite.vi"("overwrite (F)"=TRUE) -> ("overwrite?"=w242:T7)
        n55 = control-ref of="I vs Vg"() -> (w231:refnum<vi>)
        n56 = Bundle By Name(cluster=w268, "Drain Start"=w272, "Drain Stop"=w271, "Drain Step"=w270, "Drain Compliance"=w287, "Range mode"=w251, "Range"=w250) -> (w255:T5)
        n57 = call "4155C Transfer.vi"("VISA resource name in"=w257, "Gate"=w254, "Drain"=w255, "Timings"=w285, "error in (no error)"=w258, "SMU4"=w245, "sweep mode"=w278, "Panel Controls"=w244) -> ("VG"=w235:dbl[], "Outparams"=w249:T8, "VISA Resource Name out"=w284:refnum<visa-resource-name>, "IS"=w236:dbl[], "ID"=w241:dbl[], "IG"=w237:dbl[], "error out"=w222:errorcluster, "SMU4"=w246:dbl[])  [unwired: 12 in]
        n58 = Unbundle By Name(w249) -> ("V2 Step"=w248:dbl, "V2 Start"=w247:dbl, "Number of points"=w232:i32)
        n59 = call "4155C Split array.vi"("Number of VAR2 steps"=w232, "Y2 data in"=w241, "X data in"=w235, "Y1 data in"=w236, "Y3 data in"=w237, "error in (no error)"=w222) -> ("Array of clusters"=w225:cluster{"Y data in":dbl[], "X data in":dbl[]}[], "error out"=w223:errorcluster)  [unwired: 1 in]
        n60 = local write "I vs Vg"(w225) -> ()
        n61 = Absolute Value(x=w236) -> (abs(x)=w240:dbl[])
        n62 = Array Max & Min(array=w236) -> (max value=w238:dbl)  [unwired: 3 out]
        n63 = Array Max & Min(array=w237) -> (max value=w239:dbl)  [unwired: 3 out]
        n64 = local write "Is"(w238) -> ()
        n65 = Array Max & Min(array=w240) -> (max value=w233:dbl, min value=w217:dbl)  [unwired: 2 out]
        n66 = local write "Ig"(w239) -> ()
        n67 = Build Array (concatenate)(w234, w233) -> (w220:dbl[])
        n68 = call "4155C Split array.vi"("X data in"=w218, "Y1 data in"=w220) -> ("Array of clusters"=w224:cluster{"Y data in":dbl[], "X data in":dbl[]}[])  [unwired: 5 in, 1 out]
        n69 = local write "Id max vs time"(w224) -> ()
        n70 = local write "Id"(w233) -> ()
        n71 = Open/Create/Replace File(file path (use dialog)=w288, error in=w223, operation (0:open)=w242) -> (refnum out=w213:refnum<file>, error out=w211:errorcluster)  [unwired: 3 in, 1 out]
        n72 = call "4155C Make Big 2d array.vi"("1D Var1"=w235, "1d IS"=w236, "1d ID"=w241, "1d IG"=w237, "1d SMU4"=w246, "SMU4"=w245, "VAR2 START"=w247, "Number of VAR2 steps"=w232, "VAR2 STEP"=w248, "VAR1 Name"="Vg", "Decimal places in header"=i8 1, "VAR2 Name"="Vd") -> ("Header array"=w214:string[], "Data array"=w212:dbl[][])  [unwired: 14 in]
        n73 = call "4155C Config Chart Colours.vi"("Numeric"=w232, "XY Graph 2"=w231) -> ()  [unwired: 6 in]
        n74 = call "4155C Write array to file.vi"("Byte Stream File Refnum"=w213, "Header"=w214, "Data Array"=w212, "error in (no error)"=w211) -> ("dup refnum"=w210:refnum<file>, "error out"=w209:errorcluster)  [unwired: 1 in]
        n75 = Build Array (concatenate)(w215, w217) -> (w216:dbl[])
        n76 = Close File(refnum=w210, error in=w209) -> (error out=w283:errorcluster)  [unwired: 1 out]
      }
      frame "pulsedstressV" {
        w308 = 0
        n77 = Number To Decimal String(number=w299) -> (decimal integer string=w356:string)  [unwired: 1 in]
        n78 = Delete From Array(array=w348, index=0 ("Index")) -> (deleted portion=w346:string, array with subset deleted=w345:string[])  [unwired: 1 in]
        n79 = Bundle By Name(cluster=w325, "Emergency Stop"=w359) -> (w327:T2)
        n80 = VISA Write(VISA resource name=w339, write buffer=":PAGE:CHAN:MODE SWE;" ("write buffer (\"\")"), error in (no error)=w338) -> (VISA resource name out=w336:refnum<visa-resource-name>, error out=w337:errorcluster)  [unwired: 1 out]
        n81 = Concatenate Strings(w355, "-pulsedstressV-" ("Substring"), w356, w298, ".txt" ("Substring")) -> (w358:string)
        n82 = case shown="\"d\", Default" w346 {
          tunnel: [w368 w369] -> w344
          frame "s" {
            w368 = u16 0 items=["Single", "Double"] ("sweep mode")
          }
          frame "d", Default {
            w369 = u16 1 items=["Single", "Double"] ("sweep mode")
          }
        }
        n83 = Fract/Exp String To Number(string=w345) -> (number=w340:dbl[])  [unwired: 3 in, 1 out]
        n84 = String To Path(string=w358) -> (path=w354:path)
        n85 = Index Array(array=w340, index #1=0 ("Index")) -> (element #1=w317:dbl, element #2=w316:dbl, element #3=w313:dbl, element #4=w312:dbl, element #5=w311:dbl, element #6=w315:dbl)  [unwired: 5 in]
        n86 = Bundle By Name(cluster=w314, "Pulse period"=w312, "Base voltage"=w313, "Pulse width"=w311) -> (w310:T6)
        n87 = Unbundle By Name(w310) -> ("Pulse period"=w318:dbl)
        n88 = Bundle By Name(cluster=w342, "Gate Start"=w316, "Gate Stop"=w317, "Gate Step (linear only)"=0, "Gate Compliance"=w352, "Range mode"=w332, "Range"=w331) -> (w333:T4)
        n89 = call <vilib>:"compatOverwrite.vi"("overwrite (F)"=TRUE) -> ("overwrite?"=w303:T7)
        n90 = Bundle By Name(cluster=w341, "Drain Start"=w315, "Drain Stop"=w308, "Drain Step"=w308, "Drain Compliance"=w353, "Range mode"=w330, "Range"=w329) -> (w334:T5)
        n91 = call "4155C PulsedStressV.vi"("VISA resource name in"=w336, "sweep mode"=w344, "Panel Controls"=w327, "Gate"=w333, "Drain"=w334, "Timings"=w310, "error in (no error)"=w337, "SMU4"=w326) -> ("VISA Resource Name out"=w350:refnum<visa-resource-name>, "ID"=w306:dbl[], "IG"=w304:dbl[], "Outparams"=w328:T8, "error out"=w351:errorcluster)  [unwired: 3 in]
        n92 = Unbundle By Name(w328) -> ("Number of points"=w305:i32)  [unwired: 2 out]
        n93 = for {
          N: w305 -> [_]
          tunnel: [w365] -> w307 mode=indexing
          tunnel: w318 -> [w367]
          i -> [w366]
          n94 = Multiply(x=w367, y=w366) -> (x*y=w365:dbl)
        }
        n95 = Insert Into Array(array=dbl[][] [] ("Input Array"), new element=w307) -> (w319:dbl[][])  [unwired: 2 in]
        n96 = Insert Into Array(array=w319, new element=w306) -> (w324:dbl[][])  [unwired: 2 in]
        n97 = Insert Into Array(array=w324, new element=w304) -> (w323:dbl[][])  [unwired: 2 in]
        n98 = Transpose 2D Array(2D array=w323) -> (transposed array=w322:dbl[][])
        n99 = Open/Create/Replace File(file path (use dialog)=w354, error in=w351, operation (0:open)=w303) -> (refnum out=w362:refnum<file>, error out=w363:errorcluster)  [unwired: 3 in, 1 out]
        n100 = call "4155C Write array to file.vi"("Byte Stream File Refnum"=w362, "Header"=string[] ["Time /s", "Id /A", "Ig /A"], "Data Array"=w322, "error in (no error)"=w363) -> ("dup refnum"=w360:refnum<file>, "error out"=w361:errorcluster)  [unwired: 1 in]
        n101 = Close File(refnum=w360, error in=w361) -> (error out=w349:errorcluster)  [unwired: 1 out]
      }
      frame "transfer-fpp" {
        n102 = Number To Decimal String(number=w374) -> (decimal integer string=w428:string)  [unwired: 1 in]
        n103 = Bundle By Name(cluster=w404, "Emergency Stop"=w432) -> (w440:T1)
        n104 = Delete From Array(array=w419, index=0 ("Index")) -> (deleted portion=w417:string, array with subset deleted=w416:string[])  [unwired: 1 in]
        n105 = Concatenate Strings(w427, "-transferfpp-" ("Substring"), w428, w372, ".txt" ("Substring")) -> (w430:string)
        n106 = VISA Write(VISA resource name=w396, write buffer=":PAGE:CHAN:MODE SWE;" ("write buffer (\"\")"), error in (no error)=w395) -> (VISA resource name out=w393:refnum<visa-resource-name>, error out=w394:errorcluster)  [unwired: 1 out]
        n107 = case shown="\"d\", Default" w417 {
          tunnel: [w441 w442] -> w415
          frame "s" {
            w441 = u16 0 items=["Single", "Double"] ("sweep mode")
          }
          frame "d", Default {
            w442 = u16 1 items=["Single", "Double"] ("sweep mode")
          }
        }
        n108 = Fract/Exp String To Number(string=w416) -> (number=w400:dbl[])  [unwired: 3 in, 1 out]
        n109 = String To Path(string=w430) -> (path=w426:path)
        n110 = Index Array(array=w400, index #1=0 ("Index")) -> (element #1=w414:dbl, element #2=w413:dbl, element #3=w412:dbl)  [unwired: 2 in]
        n111 = Delete From Array(array=w400, length=3 ("Length"), index=0 ("Index")) -> (array with subset deleted=w398:dbl[])  [unwired: 1 out]
        n112 = Bundle By Name(cluster=w406, "Gate Start"=w414, "Gate Stop"=w413, "Gate Step (linear only)"=w412, "Gate Compliance"=w424, "Range mode"=w389, "Range"=w388) -> (w390:T4)
        n113 = Index Array(array=w398, index #1=0 ("Index")) -> (element #1=w409:dbl, element #2=w408:dbl, element #3=w407:dbl)  [unwired: 2 in]
        n114 = call <vilib>:"compatOverwrite.vi"("overwrite (F)"=TRUE) -> ("overwrite?"=w377:T7)
        n115 = Bundle By Name(cluster=w405, "Drain Start"=w409, "Drain Stop"=w408, "Drain Step"=w407, "Drain Compliance"=w425, "Range mode"=w387, "Range"=w386) -> (w391:T5)
        n116 = call "4155C Transfer-FPP.vi"("VISA resource name in"=w393, "Gate"=w390, "Drain"=w391, "Timings"=w423, "error in (no error)"=w394, "sweep mode"=w415, "Panel Controls"=w440) -> ("VG"=w431:dbl[], "Outparams"=w385:T8, "VISA Resource Name out"=w421:refnum<visa-resource-name>, "Vprobe2"=w381:dbl[], "ID"=w380:dbl[], "IG"=w379:dbl[], "Vprobe1"=w378:dbl[], "error out"=w422:errorcluster)  [unwired: 13 in]
        n117 = Unbundle By Name(w385) -> ("V2 Step"=w384:dbl, "V2 Start"=w383:dbl, "Number of points"=w382:i32)
        n118 = Open/Create/Replace File(file path (use dialog)=w426, error in=w422, operation (0:open)=w377) -> (refnum out=w437:refnum<file>, error out=w438:errorcluster)  [unwired: 3 in, 1 out]
        n119 = call "4155C Make Big 2d array FPP.vi"("1D Var1"=w431, "1d ID"=w380, "1d Vp2"=w381, "1d IG"=w379, "1d Vp1"=w378, "VAR2 START"=w383, "Number of VAR2 steps"=w382, "VAR2 STEP"=w384, "VAR1 Name"="Vg", "Decimal places in header"=i8 1, "VAR2 Name"="Vd") -> ("Header array"=w433:string[], "Data array"=w434:dbl[][])  [unwired: 15 in]
        n120 = call "4155C Write array to file.vi"("Byte Stream File Refnum"=w437, "Header"=w433, "Data Array"=w434, "error in (no error)"=w438) -> ("dup refnum"=w435:refnum<file>, "error out"=w436:errorcluster)  [unwired: 1 in]
        n121 = Close File(refnum=w435, error in=w436) -> (error out=w420:errorcluster)  [unwired: 1 out]
      }
      frame "output" {
        n122 = Number To Decimal String(number=w455) -> (decimal integer string=w504:string)  [unwired: 1 in]
        n123 = Bundle By Name(cluster=w481, "Emergency Stop"=w507) -> (w517:T1)
        n124 = Delete From Array(array=w496, index=0 ("Index")) -> (deleted portion=w494:string, array with subset deleted=w493:string[])  [unwired: 1 in]
        n125 = Concatenate Strings(w503, "-output-" ("Substring"), w504, w454, ".txt" ("Substring")) -> (w506:string)
        n126 = VISA Write(VISA resource name=w472, write buffer=":PAGE:CHAN:MODE SWE;" ("write buffer (\"\")"), error in (no error)=w469) -> (VISA resource name out=w471:refnum<visa-resource-name>, error out=w470:errorcluster)  [unwired: 1 out]
        n127 = case shown="\"d\", Default" w494 {
          tunnel: [w518 w519] -> w492
          frame "s" {
            w518 = u16 0 items=["Single", "Double"] ("sweep mode")
          }
          frame "d", Default {
            w519 = u16 1 items=["Single", "Double"] ("sweep mode")
          }
        }
        n128 = Fract/Exp String To Number(string=w493) -> (number=w475:dbl[])  [unwired: 3 in, 1 out]
        n129 = String To Path(string=w506) -> (path=w502:path)
        n130 = Index Array(array=w475, index #1=0 ("Index")) -> (element #1=w491:dbl, element #2=w490:dbl, element #3=w489:dbl)  [unwired: 2 in]
        n131 = Delete From Array(array=w475, length=3 ("Length"), index=0 ("Index")) -> (array with subset deleted=w474:dbl[])  [unwired: 1 out]
        n132 = control-ref of="I vs Vd"() -> (w445:refnum<vi>)
        n133 = Bundle By Name(cluster=w483, "Gate Start"=w491, "Gate Stop"=w490, "Gate Step (linear only)"=w489, "Gate Compliance"=w500, "Range mode"=w467, "Range"=w466) -> (w516:T4)
        n134 = Index Array(array=w474, index #1=0 ("Index")) -> (element #1=w486:dbl, element #2=w485:dbl, element #3=w484:dbl)  [unwired: 2 in]
        n135 = call <vilib>:"compatOverwrite.vi"("overwrite (F)"=TRUE) -> ("overwrite?"=w459:T7)
        n136 = Bundle By Name(cluster=w482, "Drain Start"=w486, "Drain Stop"=w485, "Drain Step"=w484, "Drain Compliance"=w501, "Range mode"=w465, "Range"=w468) -> (w515:T5)
        n137 = call "4155C Output.vi"("VISA resource name in"=w471, "Gate"=w516, "Drain"=w515, "Timings"=w499, "error in (no error)"=w470, "SMU4"=w461, "sweep mode"=w492, "Panel controls"=w517) -> ("VD"=w452:dbl[], "Outparams"=w463:T8, "VISA Resource Name out"=w498:refnum<visa-resource-name>, "IS"=w451:dbl[], "ID"=w450:dbl[], "IG"=w449:dbl[], "error out"=w447:errorcluster, "SMU4"=w460:dbl[])  [unwired: 12 in]
        n138 = Unbundle By Name(w463) -> ("V2 Step"=w464:dbl, "V2 Start"=w462:dbl, "Number of points"=w444:i32)
        n139 = call "4155C Split array.vi"("Number of VAR2 steps"=w444, "Y2 data in"=w450, "X data in"=w452, "Y1 data in"=w451, "Y3 data in"=w449, "error in (no error)"=w447) -> ("Array of clusters"=w448:cluster{"Y data in":dbl[], "X data in":dbl[]}[], "error out"=w446:errorcluster)  [unwired: 1 in]
        n140 = local write "I vs Vd"(w448) -> ()
        n141 = call "4155C Config Chart Colours.vi"("Numeric"=w444, "XY Graph 2"=w445) -> ()  [unwired: 6 in]
        n142 = Open/Create/Replace File(file path (use dialog)=w502, error in=w446, operation (0:open)=w459) -> (refnum out=w512:refnum<file>, error out=w513:errorcluster)  [unwired: 3 in, 1 out]
        n143 = call "4155C Make Big 2d array.vi"("1D Var1"=w452, "1d IS"=w451, "1d ID"=w450, "1d IG"=w449, "1d SMU4"=w460, "SMU4"=w461, "VAR2 START"=w462, "Number of VAR2 steps"=w444, "VAR2 STEP"=w464, "VAR1 Name"="Vd", "Decimal places in header"=i8 1, "VAR2 Name"="Vg") -> ("Header array"=w508:string[], "Data array"=w509:dbl[][])  [unwired: 14 in]
        n144 = call "4155C Write array to file.vi"("Byte Stream File Refnum"=w512, "Header"=w508, "Data Array"=w509, "error in (no error)"=w513) -> ("dup refnum"=w510:refnum<file>, "error out"=w511:errorcluster)  [unwired: 1 in]
        n145 = Close File(refnum=w510, error in=w511) -> (error out=w497:errorcluster)  [unwired: 1 out]
      }
      frame "output-fpp" {
        n146 = Number To Decimal String(number=w523) -> (decimal integer string=w577:string)  [unwired: 1 in]
        n147 = Bundle By Name(cluster=w553, "Emergency Stop"=w580) -> (w590:T1)
        n148 = Delete From Array(array=w568, index=0 ("Index")) -> (deleted portion=w566:string, array with subset deleted=w565:string[])  [unwired: 1 in]
        n149 = VISA Write(VISA resource name=w544, write buffer=":PAGE:CHAN:MODE SWE;" ("write buffer (\"\")"), error in (no error)=w541) -> (VISA resource name out=w543:refnum<visa-resource-name>, error out=w542:errorcluster)  [unwired: 1 out]
        n150 = Concatenate Strings(w576, "-outputfpp-" ("Substring"), w577, w522, ".txt" ("Substring")) -> (w579:string)
        n151 = case shown="\"d\", Default" w566 {
          tunnel: [w591 w592] -> w564
          frame "s" {
            w591 = u16 0 items=["Single", "Double"] ("sweep mode")
          }
          frame "d", Default {
            w592 = u16 1 items=["Single", "Double"] ("sweep mode")
          }
        }
        n152 = Fract/Exp String To Number(string=w565) -> (number=w547:dbl[])  [unwired: 3 in, 1 out]
        n153 = String To Path(string=w579) -> (path=w575:path)
        n154 = Index Array(array=w547, index #1=0 ("Index")) -> (element #1=w563:dbl, element #2=w562:dbl, element #3=w561:dbl)  [unwired: 2 in]
        n155 = Delete From Array(array=w547, length=3 ("Length"), index=0 ("Index")) -> (array with subset deleted=w546:dbl[])  [unwired: 1 out]
        n156 = Bundle By Name(cluster=w555, "Gate Start"=w563, "Gate Stop"=w562, "Gate Step (linear only)"=w561, "Gate Compliance"=w573, "Range mode"=w539, "Range"=w538) -> (w589:T4)
        n157 = Index Array(array=w546, index #1=0 ("Index")) -> (element #1=w558:dbl, element #2=w557:dbl, element #3=w556:dbl)  [unwired: 2 in]
        n158 = call <vilib>:"compatOverwrite.vi"("overwrite (F)"=TRUE) -> ("overwrite?"=w527:T7)
        n159 = Bundle By Name(cluster=w554, "Drain Start"=w558, "Drain Stop"=w557, "Drain Step"=w556, "Drain Compliance"=w574, "Range mode"=w537, "Range"=w540) -> (w588:T5)
        n160 = call "4155C Output-FPP.vi"("VISA resource name in"=w543, "Gate"=w589, "Drain"=w588, "Timings"=w572, "error in (no error)"=w542, "sweep mode"=w564, "Panel controls"=w590) -> ("VD"=w532:dbl[], "Outparams"=w535:T8, "VISA Resource Name out"=w570:refnum<visa-resource-name>, "Vprobe2"=w531:dbl[], "ID"=w530:dbl[], "IG"=w529:dbl[], "Vprobe1"=w528:dbl[], "error out"=w571:errorcluster)  [unwired: 13 in]
        n161 = Unbundle By Name(w535) -> ("V2 Step"=w536:dbl, "V2 Start"=w534:dbl, "Number of points"=w533:i32)
        n162 = Open/Create/Replace File(file path (use dialog)=w575, error in=w571, operation (0:open)=w527) -> (refnum out=w585:refnum<file>, error out=w586:errorcluster)  [unwired: 3 in, 1 out]
        n163 = call "4155C Make Big 2d array FPP.vi"("1D Var1"=w532, "1d ID"=w530, "1d Vp2"=w531, "1d IG"=w529, "1d Vp1"=w528, "VAR2 START"=w534, "Number of VAR2 steps"=w533, "VAR2 STEP"=w536, "VAR1 Name"="Vd", "Decimal places in header"=i8 1, "VAR2 Name"="Vg") -> ("Header array"=w581:string[], "Data array"=w582:dbl[][])  [unwired: 15 in]
        n164 = call "4155C Write array to file.vi"("Byte Stream File Refnum"=w585, "Header"=w581, "Data Array"=w582, "error in (no error)"=w586) -> ("dup refnum"=w583:refnum<file>, "error out"=w584:errorcluster)  [unwired: 1 in]
        n165 = Close File(refnum=w583, error in=w584) -> (error out=w569:errorcluster)  [unwired: 1 out]
      }
      frame "itime" {
        n166 = Delete From Array(array=w608, index=0 ("Index")) -> (deleted portion=w609:string)  [unwired: 1 in, 1 out]
        n167 = case shown="\"l\"" w609 {
          tunnel: w607 -> [w613 w615 w618]
          tunnel: [w612 w614 w617] -> w600
          frame "s" {
            w611 = u32 0 items=["short  ", "medium  ", "long  "] ("integration time 2")
            n168 = Bundle By Name(cluster=w613, "integration time"=w611) -> (w612:T6)
          }
          frame "m", Default {
            w616 = u32 1 items=["short  ", "medium  ", "long  "] ("integration time 2")
            n169 = Bundle By Name(cluster=w615, "integration time"=w616) -> (w614:T6)
          }
          frame "l" {
            w619 = u32 2 items=["short  ", "medium  ", "long  "] ("integration time 2")
            n170 = Bundle By Name(cluster=w618, "integration time"=w619) -> (w617:T6)
          }
        }
      }
      frame "pulsed" {
        n171 = Delete From Array(array=w636, index=0 ("Index")) -> (deleted portion=w637:string, array with subset deleted=w624:string[])  [unwired: 1 in]
        n172 = case shown="\"on\", Default" w637 {
          tunnel: w635 -> [w647 w650]
          tunnel: [w646 w649] -> w628
          tunnel: w624 -> [w644 _]
          frame "on", Default {
            w645 = u16 1 items=["Continuous", "Pulsed"] ("sweep method")
            n173 = Fract/Exp String To Number(string=w644) -> (number=w642:dbl[])  [unwired: 3 in, 1 out]
            n174 = Index Array(array=w642, index #1=0 ("Index")) -> (element #1=w641:dbl, element #2=w640:dbl, element #3=w639:dbl)  [unwired: 2 in]
            n175 = Bundle By Name(cluster=w647, "sweep method"=w645, "Pulse period"=w641, "Base voltage"=w640, "Pulse width"=w639) -> (w646:T6)
          }
          frame "off" {
            w648 = u16 0 items=["Continuous", "Pulsed"] ("sweep method")
            n176 = Bundle By Name(cluster=w650, "sweep method"=w648) -> (w649:T6)
          }
        }
      }
      frame "gaterangemode" {
        n177 = Delete From Array(array=w665, index=0 ("Index")) -> (deleted portion=w666:string)  [unwired: 1 in, 1 out]
        n178 = case shown="\"f\"" w666 {
          tunnel: [w668 w669 w670] -> w655
          frame "a", Default {
            w668 = u16 0 items=["Auto", "Limited", "Fixed"] ("Gate Range\nmode 2")
          }
          frame "f" {
            w669 = u16 2 items=["Auto", "Limited", "Fixed"] ("Gate Range\nmode 2")
          }
          frame "l" {
            w670 = u16 1 items=["Auto", "Limited", "Fixed"] ("Gate Range\nmode 2")
          }
        }
      }
      frame "gaterange" {
        (unwired) u8 11 items=["10fA  ", "100fA  ", "1nA  ", "10nA", "100nA", "1uA", "10uA", "100uA", "1mA", "10mA", "100mA", "1A"] ("Gate Range 2")
        n179 = Delete From Array(array=w692, index=0 ("Index")) -> (deleted portion=w682:string)  [unwired: 1 in, 1 out]
        n180 = Scan Value(string=w682, format string="") -> (value=w680:dbl)  [unwired: 1 in, 1 out]
        n181 = Logarithm Base 10(1:w680) -> (0:w679:dbl)
        n182 = Round To Nearest(number=w679) -> (nearest integer value=w678:dbl)
        n183 = Add(x=w678, y=11.0) -> (x+y=w676:dbl)
        n184 = To Unsigned Byte Integer(number=w676) -> (unsigned 8bit integer=w675:u8)
      }
      frame "drainrange" {
        (unwired) u8 11 items=["10fA  ", "100fA  ", "1nA  ", "10nA", "100nA", "1uA", "10uA", "100uA", "1mA", "10mA", "100mA", "1A"] ("Gate Range 2")
        n185 = Delete From Array(array=w715, index=0 ("Index")) -> (deleted portion=w706:string)  [unwired: 1 in, 1 out]
        n186 = Scan Value(string=w706, format string="") -> (value=w704:dbl)  [unwired: 1 in, 1 out]
        n187 = Logarithm Base 10(1:w704) -> (0:w703:dbl)
        n188 = Round To Nearest(number=w703) -> (nearest integer value=w702:dbl)
        n189 = Add(x=w702, y=11.0) -> (x+y=w700:dbl)
        n190 = To Unsigned Byte Integer(number=w700) -> (unsigned 8bit integer=w699:u8)
      }
      frame "drainrangemode" {
        n191 = Delete From Array(array=w731, index=0 ("Index")) -> (deleted portion=w732:string)  [unwired: 1 in, 1 out]
        n192 = case shown="\"f\"" w732 {
          tunnel: [w734 w735 w736] -> w721
          frame "a", Default {
            w734 = u16 0 items=["Auto", "Limited", "Fixed"] ("Gate Range\nmode 2")
          }
          frame "f" {
            w735 = u16 2 items=["Auto", "Limited", "Fixed"] ("Gate Range\nmode 2")
          }
          frame "l" {
            w736 = u16 1 items=["Auto", "Limited", "Fixed"] ("Gate Range\nmode 2")
          }
        }
      }
      frame "Error", Default {
      }
      frame "logfile" {
        n193 = Number To Decimal String(number=w755) -> (decimal integer string=w790:string)  [unwired: 1 in]
        n194 = Concatenate Strings(w789, "logfile" ("Substring"), w790, w753, ".txt" ("Substring")) -> (w787:string)
        n195 = String To Path(string=w787) -> (path=w760:path)
        n196 = Unbundle(w786) -> ("integration time"=w785:u32, "Short/Long integration time"=w784:dbl, "hold time (sec)"=w783:dbl, "delay time (sec)"=w782:dbl, "Step Time (0 disables)"=w781:dbl, "sweep method"=w780:u16, "Pulse period"=w779:dbl, "Base voltage"=w778:dbl, "Pulse width"=w777:dbl)
        n197 = Build Array(w785, w784, w783, w782, w781, w780, w779, w778, w777, w771, w772, w773, w774, w775, w776) -> (w764:dbl[])
        n198 = Insert Into Array(array=dbl[][] [] ("Input Array"), new element=w764) -> (w763:dbl[][])  [unwired: 2 in]
        n199 = call <vilib>:"compatOverwrite.vi"("overwrite (F)"=TRUE) -> ("overwrite?"=w758:T7)
        n200 = Open/Create/Replace File(file path (use dialog)=w760, error in=w762, operation (0:open)=w758) -> (refnum out=w768:refnum<file>, error out=w767:errorcluster)  [unwired: 3 in, 1 out]
        n201 = call "4155C Write array to file.vi"("Byte Stream File Refnum"=w768, "Header"=string[] ["Int Time", "Short/Long Itime", "Hold time", "Delay time", "Step time", "Sweep method", "Pulse period", "Base Voltage", "Pulse width", "Drain compliance", "Gate compliance", "Gate range mode", "Gate range", "S/D range mode", "S/D range"], "Data Array"=w763, "error in (no error)"=w767) -> ("dup refnum"=w770:refnum<file>, "error out"=w769:errorcluster)  [unwired: 1 in]
        n202 = Close File(refnum=w770, error in=w769) -> (error out=w761:errorcluster)  [unwired: 1 out]
      }
      frame "sample" {
        n203 = Number To Decimal String(number=w796) -> (decimal integer string=w844:string)  [unwired: 1 in]
        n204 = Fract/Exp String To Number(string=w841) -> (number=w802:dbl[])  [unwired: 3 in, 1 out]
        n205 = Concatenate Strings(w819, "-sample-" ("Substring"), w844, w794, ".txt" ("Substring")) -> (w842:string)
        n206 = String To Path(string=w842) -> (path=w823:path)
        n207 = Index Array(array=w802, index=0 ("Index")) -> (element=w839:dbl)
        n208 = Index Array(array=w802, index=2 ("Index")) -> (element=w835:dbl)
        n209 = Index Array(array=w802, index=3 ("Index")) -> (element=w804:dbl)
        n210 = Index Array(array=w802, index=4 ("Index")) -> (element=w801:dbl)
        n211 = call "4155C Config Sampling Measurements.vi"("Sampling interval"=w801, "Sample time"=w804, "Display on/off"=TRUE, "Timings"=w810, "Num Points"=w835, "error in (no error)"=w846, "Drain Compliance"=w845, "Gate Compliance"=w820, "VISA session"=w847) -> ("error out"=w848:errorcluster, "dup VISA resource name"=w849:refnum<visa-resource-name>)  [unwired: 1 in]
        n212 = Index Array(array=w802, index=1 ("Index")) -> (element=w836:dbl)
        n213 = call "4155C Take Sample.vi"("Emergency Stop"=w816, "error in (no error)"=w848, "Vd"=w836, "Vg"=w839, "VISA resource name in"=w849) -> ("error out"=w814:errorcluster, "Id"=w851:dbl[], "Ig"=w825:dbl[], "VISA Resource Name out"=w812:refnum<visa-resource-name>, "Is"=w850:dbl[], "Time"=w829:dbl[])  [unwired: 1 in]
        n214 = Insert Into Array(array=dbl[][] [] ("Input Array"), new element=w829) -> (w828:dbl[][])  [unwired: 2 in]
        n215 = Insert Into Array(array=w828, new element=w825) -> (w827:dbl[][])  [unwired: 2 in]
        n216 = Insert Into Array(array=w827, new element=w851) -> (w826:dbl[][])  [unwired: 2 in]
        n217 = VISA Write(VISA resource name=w812, write buffer=":DISP ON" ("write buffer (\"\")"), error in (no error)=w814) -> (VISA resource name out=w811:refnum<visa-resource-name>, error out=w813:errorcluster)  [unwired: 1 out]
        n218 = Insert Into Array(array=w826, new element=w850) -> (w818:dbl[][])  [unwired: 2 in]
        n219 = Transpose 2D Array(2D array=w818) -> (transposed array=w817:dbl[][])
        n220 = call <vilib>:"compatOverwrite.vi"("overwrite (F)"=TRUE) -> ("overwrite?"=w799:T7)
        n221 = Open/Create/Replace File(file path (use dialog)=w823, error in=w813, operation (0:open)=w799) -> (refnum out=w832:refnum<file>, error out=w831:errorcluster)  [unwired: 3 in, 1 out]
        n222 = call "4155C Write array to file.vi"("Byte Stream File Refnum"=w832, "Header"=string[] ["Time /s", "Ig /A", "Id /A", "Is /A"], "Data Array"=w817, "error in (no error)"=w831) -> ("dup refnum"=w834:refnum<file>, "error out"=w833:errorcluster)  [unwired: 1 in]
        n223 = Close File(refnum=w834, error in=w833) -> (error out=w821:errorcluster)  [unwired: 1 out]
      }
      frame "samplei" {
        n224 = Number To Decimal String(number=w855) -> (decimal integer string=w907:string)  [unwired: 1 in]
        n225 = Fract/Exp String To Number(string=w904) -> (number=w871:dbl[])  [unwired: 3 in, 1 out]
        n226 = Concatenate Strings(w886, "-samplei-" ("Substring"), w907, w854, ".txt" ("Substring")) -> (w905:string)
        n227 = String To Path(string=w905) -> (path=w889:path)
        n228 = Index Array(array=w871, index=4 ("Index")) -> (element=w865:dbl)
        n229 = Index Array(array=w871, index=3 ("Index")) -> (element=w866:dbl)
        n230 = Index Array(array=w871, index=1 ("Index")) -> (element=w868:dbl)
        n231 = Index Array(array=w871, index=0 ("Index")) -> (element=w869:dbl)
        n232 = Index Array(array=w871, index=2 ("Index")) -> (element=w867:dbl)
        n233 = call "4155C Config SamplingI Measurements.vi"("Sample time"=w867, "Display on/off"=TRUE, "Timings"=w878, "Num Points"=w868, "error in (no error)"=w909, "Sampling interval"=w866, "VISA session"=w910) -> ("error out"=w911:errorcluster, "dup VISA resource name"=w912:refnum<visa-resource-name>)  [unwired: 3 in]
        n234 = call "4155C Take SampleI.vi"("Emergency Stop"=w883, "error in (no error)"=w911, "Idg 2"=w869, "Vdg compliance 2"=w865, "VISA resource name in"=w912) -> ("error out"=w881:errorcluster, "Idg"=w914:dbl[], "Vdg"=w891:dbl[], "VISA Resource Name out"=w879:refnum<visa-resource-name>, "Is"=w913:dbl[], "Time"=w895:dbl[])  [unwired: 1 in]
        n235 = Insert Into Array(array=dbl[][] [] ("Input Array"), new element=w895) -> (w894:dbl[][])  [unwired: 2 in]
        n236 = Insert Into Array(array=w894, new element=w891) -> (w893:dbl[][])  [unwired: 2 in]
        n237 = Insert Into Array(array=w893, new element=w914) -> (w892:dbl[][])  [unwired: 2 in]
        n238 = VISA Write(VISA resource name=w879, write buffer=":DISP ON" ("write buffer (\"\")"), error in (no error)=w881) -> (VISA resource name out=w864:refnum<visa-resource-name>, error out=w880:errorcluster)  [unwired: 1 out]
        n239 = Insert Into Array(array=w892, new element=w913) -> (w885:dbl[][])  [unwired: 2 in]
        n240 = Transpose 2D Array(2D array=w885) -> (transposed array=w884:dbl[][])
        n241 = call <vilib>:"compatOverwrite.vi"("overwrite (F)"=TRUE) -> ("overwrite?"=w859:T7)
        n242 = Open/Create/Replace File(file path (use dialog)=w889, error in=w880, operation (0:open)=w859) -> (refnum out=w898:refnum<file>, error out=w897:errorcluster)  [unwired: 3 in, 1 out]
        n243 = call "4155C Write array to file.vi"("Byte Stream File Refnum"=w898, "Header"=string[] ["Time /s", "Vdg /V", "Idg /A", "Is /A"], "Data Array"=w884, "error in (no error)"=w897) -> ("dup refnum"=w900:refnum<file>, "error out"=w899:errorcluster)  [unwired: 1 in]
        n244 = Close File(refnum=w900, error in=w899) -> (error out=w862:errorcluster)  [unwired: 1 out]
        n245 = VISA Write(VISA resource name=w864, write buffer=";:PAGE:SCON:STAN OFF;:PAGE:CHAN:VSU2:DIS;" ("write buffer (\"\")"), error in (no error)=w862) -> (VISA resource name out=w860:refnum<visa-resource-name>, error out=w861:errorcluster)  [unwired: 1 out]
      }
      frame "#" {
        n246 = VISA Write(VISA resource name=w923, write buffer=":DISP ON" ("write buffer (\"\")"), error in (no error)=w922) -> (VISA resource name out=w921:refnum<visa-resource-name>, error out=w920:errorcluster)  [unwired: 1 out]
      }
      frame "stressV" {
        n247 = Number To Decimal String(number=w935) -> (decimal integer string=w976:string)  [unwired: 1 in]
        n248 = Fract/Exp String To Number(string=w973) -> (number=w946:dbl[])  [unwired: 3 in, 1 out]
        n249 = Concatenate Strings(w960, "-stressV-" ("Substring"), w976, w934, ".txt" ("Substring")) -> (w974:string)
        n250 = String To Path(string=w974) -> (path=w964:path)
        n251 = Index Array(array=w946, index=3 ("Index")) -> (element=w943:dbl)
        n252 = Index Array(array=w946, index=1 ("Index")) -> (element=w941:dbl)
        n253 = Index Array(array=w946, index=0 ("Index")) -> (element=w940:dbl)
        n254 = Index Array(array=w946, index=4 ("Index")) -> (element=w945:dbl)
        n255 = Index Array(array=w946, index=2 ("Index")) -> (element=w942:dbl)
        n256 = call "4155C Config V Stress.vi"("VISA session"=w979, "ID compliance"=w943, "VD"=w941, "VG"=w940, "IG compliance"=w942, "error in (no error)"=w978, "Display on/off"=TRUE) -> ("dup VISA resource name"=w981:refnum<visa-resource-name>, "error out"=w980:errorcluster)
        n257 = call "4155C Apply Stress.vi"("error in (no error)"=w980, "Duration"=w945, "Emergency Stop"=w959, "VISA resource name in"=w981) -> ("error out"=w957:errorcluster, "VISA Resource Name out"=w955:refnum<visa-resource-name>)
        n258 = VISA Write(VISA resource name=w955, write buffer=":DISP ON" ("write buffer (\"\")"), error in (no error)=w957) -> (VISA resource name out=w954:refnum<visa-resource-name>, error out=w956:errorcluster)  [unwired: 1 out]
        n259 = call <vilib>:"compatOverwrite.vi"("overwrite (F)"=TRUE) -> ("overwrite?"=w939:T7)
        n260 = Open/Create/Replace File(file path (use dialog)=w964, error in=w956, operation (0:open)=w939) -> (refnum out=w967:refnum<file>, error out=w966:errorcluster)  [unwired: 3 in, 1 out]
        n261 = call "4155C Write array to file.vi"("Byte Stream File Refnum"=w967, "Header"=string[] ["V stress completed successfully", ""], "error in (no error)"=w966) -> ("dup refnum"=w969:refnum<file>, "error out"=w968:errorcluster)  [unwired: 2 in]
        n262 = Close File(refnum=w969, error in=w968) -> (error out=w962:errorcluster)  [unwired: 1 out]
      }
      frame "stressI" {
        n263 = Number To Decimal String(number=w985) -> (decimal integer string=w1022:string)  [unwired: 1 in]
        n264 = Fract/Exp String To Number(string=w1019) -> (number=w994:dbl[])  [unwired: 3 in, 1 out]
        n265 = Concatenate Strings(w1006, "-stressI-" ("Substring"), w1022, w984, ".txt" ("Substring")) -> (w1020:string)
        n266 = String To Path(string=w1020) -> (path=w1010:path)
        n267 = Index Array(array=w994, index=1 ("Index")) -> (element=w990:dbl)
        n268 = Index Array(array=w994, index=0 ("Index")) -> (element=w991:dbl)
        n269 = call "4155C Config I Stress.vi"("VISA session"=w1025, "IDG"=w991, "VDG compliance"=w990, "error in (no error)"=w1024, "Display on/off"=TRUE) -> ("dup VISA resource name"=w1027:refnum<visa-resource-name>, "error out"=w1026:errorcluster)
        n270 = Index Array(array=w994, index=2 ("Index")) -> (element=w992:dbl)
        n271 = call "4155C Apply Stress.vi"("error in (no error)"=w1026, "Duration"=w992, "Emergency Stop"=w1005, "VISA resource name in"=w1027) -> ("error out"=w1003:errorcluster, "VISA Resource Name out"=w1001:refnum<visa-resource-name>)
        n272 = VISA Write(VISA resource name=w1001, write buffer=":DISP ON" ("write buffer (\"\")"), error in (no error)=w1003) -> (VISA resource name out=w1000:refnum<visa-resource-name>, error out=w1002:errorcluster)  [unwired: 1 out]
        n273 = call <vilib>:"compatOverwrite.vi"("overwrite (F)"=TRUE) -> ("overwrite?"=w989:T7)
        n274 = Open/Create/Replace File(file path (use dialog)=w1010, error in=w1002, operation (0:open)=w989) -> (refnum out=w1013:refnum<file>, error out=w1012:errorcluster)  [unwired: 3 in, 1 out]
        n275 = call "4155C Write array to file.vi"("Byte Stream File Refnum"=w1013, "Header"=string[] ["I stress completed successfully", ""], "error in (no error)"=w1012) -> ("dup refnum"=w1015:refnum<file>, "error out"=w1014:errorcluster)  [unwired: 2 in]
        n276 = Close File(refnum=w1015, error in=w1014) -> (error out=w1008:errorcluster)  [unwired: 1 out]
      }
      frame "vsu2pulse" {
        n277 = Number To Decimal String(number=w1031) -> (decimal integer string=w1066:string)  [unwired: 1 in]
        n278 = Fract/Exp String To Number(string=w1063) -> (number=w1039:dbl[])  [unwired: 3 in, 1 out]
        n279 = Concatenate Strings(w1051, "-vsu2-" ("Substring"), w1066, w1030, ".txt" ("Substring")) -> (w1064:string)
        n280 = String To Path(string=w1064) -> (path=w1055:path)
        n281 = Index Array(array=w1039, index=1 ("Index")) -> (element=w1038:dbl)
        n282 = Index Array(array=w1039, index=0 ("Index")) -> (element=w1036:dbl)
        n283 = call "4155C Config VSU2 Stress.vi"("error in (no error)"=w1068, "VSU2"=w1036, "Display on/off"=TRUE, "VISA session"=w1069) -> ("error out"=w1070:errorcluster, "dup VISA resource name"=w1071:refnum<visa-resource-name>)
        n284 = call "4155C Apply Stress.vi"("error in (no error)"=w1070, "Duration"=w1038, "Emergency Stop"=w1050, "VISA resource name in"=w1071) -> ("error out"=w1048:errorcluster, "VISA Resource Name out"=w1046:refnum<visa-resource-name>)
        n285 = VISA Write(VISA resource name=w1046, write buffer=":DISP ON" ("write buffer (\"\")"), error in (no error)=w1048) -> (VISA resource name out=w1045:refnum<visa-resource-name>, error out=w1047:errorcluster)  [unwired: 1 out]
        n286 = call <vilib>:"compatOverwrite.vi"("overwrite (F)"=TRUE) -> ("overwrite?"=w1035:T7)
        n287 = Open/Create/Replace File(file path (use dialog)=w1055, error in=w1047, operation (0:open)=w1035) -> (refnum out=w1058:refnum<file>, error out=w1057:errorcluster)  [unwired: 3 in, 1 out]
        n288 = call "4155C Write array to file.vi"("Byte Stream File Refnum"=w1058, "Header"=string[] ["VSU2 pulse completed successfully", ""], "error in (no error)"=w1057) -> ("dup refnum"=w1060:refnum<file>, "error out"=w1059:errorcluster)  [unwired: 2 in]
        n289 = Close File(refnum=w1060, error in=w1059) -> (error out=w1053:errorcluster)  [unwired: 1 out]
      }
      frame "sample-fpp" {
        w1086 = string[] ["Time /s", "Id VgVd /A", "Ig VgVd /A", "Vp1 VgVd /V", "Vp2 VgVd /V"] ("Header")
        w1090 = "%d" ("format string")
        n290 = Number To Decimal String(number=w1075) -> (decimal integer string=w1138:string)  [unwired: 1 in]
        n291 = Fract/Exp String To Number(string=w1135) -> (number=w1123:dbl[])  [unwired: 3 in, 1 out]
        n292 = Concatenate Strings(w1129, "-samplefpp-" ("Substring"), w1138, w1074, ".txt" ("Substring")) -> (w1136:string)
        n293 = String To Path(string=w1136) -> (path=w1098:path)
        n294 = Index Array(array=w1123, index=0 ("Index")) -> (element=w1084:dbl)
        n295 = Index Array(array=w1123, index=1 ("Index")) -> (element=w1083:dbl)
        n296 = Index Array(array=w1123, index=2 ("Index")) -> (element=w1131:dbl)
        n297 = Index Array(array=w1123, index=3 ("Index")) -> (element=w1121:dbl)
        n298 = call "4155C Config Sampling Measurements FPP.vi"("VISA session"=w1141, "Num Points"=w1131, "Vg"=w1084, "Display on/off"=TRUE, "Gate Compliance"=w1130, "Drain Compliance"=w1139, "Standby"="Standby", "error in (no error)"=w1140, "Timings"=w1128, "Vd"=w1083, "Sample time"=w1121) -> ("dup VISA resource name"=w1100:refnum<visa-resource-name>, "error out"=w1099:errorcluster)  [unwired: 3 in]
        n299 = Number To Decimal String(number=w1084) -> (decimal integer string=w1110:string)  [unwired: 1 in]
        n300 = call "4155C Take Sample FPP.vi"("VISA resource name in"=w1100, "error in (no error)"=w1099, "Emergency Stop"=w1101) -> ("Time"=w1105:dbl[], "Vp1"=w1115:dbl[], "VISA Resource Name out"=w1081:refnum<visa-resource-name>, "Ig"=w1103:dbl[], "Id"=w1104:dbl[], "Vp2"=w1113:dbl[], "error out"=w1102:errorcluster)  [unwired: 10 in]
        n301 = Insert Into Array(array=dbl[][] [] ("Input Array"), new element=w1105) -> (w1119:dbl[][])  [unwired: 2 in]
        n302 = Number To Decimal String(number=w1083) -> (decimal integer string=w1108:string)  [unwired: 1 in]
        n303 = Insert Into Array(array=w1119, new element=w1104) -> (w1118:dbl[][])  [unwired: 2 in]
        n304 = Concatenate Strings("(Vg = " ("Substring"), w1110, "V, Vd = " ("Substring"), w1108, "V)" ("Substring")) -> (w1106:string)
        n305 = Insert Into Array(array=w1118, new element=w1103) -> (w1117:dbl[][])  [unwired: 2 in]
        n306 = Insert Into Array(array=w1117, new element=w1115) -> (w1114:dbl[][])  [unwired: 2 in]
        n307 = Insert Into Array(array=w1114, new element=w1113) -> (w1082:dbl[][])  [unwired: 2 in]
        n308 = call <vilib>:"compatOverwrite.vi"("overwrite (F)"=TRUE) -> ("overwrite?"=w1079:T7)
        n309 = Open/Create/Replace File(file path (use dialog)=w1098, error in=w1102, operation (0:open)=w1079) -> (refnum out=w1095:refnum<file>, error out=w1096:errorcluster)  [unwired: 3 in, 1 out]
        n310 = Array To Spreadsheet String(array=w1086, 3:w1090) -> (spreadsheet string=w1092:string)  [unwired: 1 in]
        n311 = Transpose 2D Array(2D array=w1082) -> (transposed array=w1112:dbl[][])
        n312 = Search and Replace String(replace all?=TRUE ("replace all? (F)"), input string=w1092, search string="VgVd", replace string=w1106) -> (result string=w1088:string)  [unwired: 4 in, 3 out]
        n313 = Spreadsheet String To Array(format string=w1090, spreadsheet string=w1088, array type (2D Dbl)=w1086) -> (array=w1087:string[])  [unwired: 1 in]
        n314 = call "4155C Write array to file.vi"("Byte Stream File Refnum"=w1095, "Header"=w1087, "Data Array"=w1112, "error in (no error)"=w1096) -> ("dup refnum"=w1093:refnum<file>, "error out"=w1094:errorcluster)  [unwired: 1 in]
        n315 = Close File(refnum=w1093, error in=w1094) -> (error out=w1080:errorcluster)  [unwired: 1 out]
      }
      frame "resample-fpp" {
        w1158 = string[] ["Time /s", "Id VgVd /A", "Ig VgVd /A", "Vp1 VgVd /V", "Vp2 VgVd /V"] ("Header")
        w1162 = "%d" ("format string")
        n316 = Number To Decimal String(number=w1144) -> (decimal integer string=w1202:string)  [unwired: 1 in]
        n317 = Fract/Exp String To Number(string=w1199) -> (number=w1151:dbl[])  [unwired: 3 in, 1 out]
        n318 = Concatenate Strings(w1195, "-resamplefpp-" ("Substring"), w1202, w1145, ".txt" ("Substring")) -> (w1200:string)
        n319 = String To Path(string=w1200) -> (path=w1170:path)
        n320 = Index Array(array=w1151, index=0 ("Index")) -> (element=w1157:dbl)
        n321 = Index Array(array=w1151, index=1 ("Index")) -> (element=w1156:dbl)
        n322 = Number To Decimal String(number=w1157) -> (decimal integer string=w1180:string)  [unwired: 1 in]
        n323 = call "4155C Take Sample FPP.vi"("VISA resource name in"=w1153, "error in (no error)"=w1152, "Emergency Stop"=w1171) -> ("Time"=w1175:dbl[], "Vp1"=w1185:dbl[], "VISA Resource Name out"=w1155:refnum<visa-resource-name>, "Ig"=w1173:dbl[], "Id"=w1174:dbl[], "Vp2"=w1183:dbl[], "error out"=w1172:errorcluster)  [unwired: 10 in]
        n324 = Insert Into Array(array=dbl[][] [] ("Input Array"), new element=w1175) -> (w1189:dbl[][])  [unwired: 2 in]
        n325 = Number To Decimal String(number=w1156) -> (decimal integer string=w1178:string)  [unwired: 1 in]
        n326 = Insert Into Array(array=w1189, new element=w1174) -> (w1188:dbl[][])  [unwired: 2 in]
        n327 = Concatenate Strings("(Vg = " ("Substring"), w1180, "V, Vd = " ("Substring"), w1178, "V)" ("Substring")) -> (w1176:string)
        n328 = Insert Into Array(array=w1188, new element=w1173) -> (w1187:dbl[][])  [unwired: 2 in]
        n329 = Insert Into Array(array=w1187, new element=w1185) -> (w1184:dbl[][])  [unwired: 2 in]
        n330 = Insert Into Array(array=w1184, new element=w1183) -> (w1150:dbl[][])  [unwired: 2 in]
        n331 = call <vilib>:"compatOverwrite.vi"("overwrite (F)"=TRUE) -> ("overwrite?"=w1149:T7)
        n332 = Open/Create/Replace File(file path (use dialog)=w1170, error in=w1172, operation (0:open)=w1149) -> (refnum out=w1167:refnum<file>, error out=w1168:errorcluster)  [unwired: 3 in, 1 out]
        n333 = Array To Spreadsheet String(array=w1158, 3:w1162) -> (spreadsheet string=w1164:string)  [unwired: 1 in]
        n334 = Transpose 2D Array(2D array=w1150) -> (transposed array=w1182:dbl[][])
        n335 = Search and Replace String(replace all?=TRUE ("replace all? (F)"), input string=w1164, search string="VgVd", replace string=w1176) -> (result string=w1160:string)  [unwired: 4 in, 3 out]
        n336 = Spreadsheet String To Array(format string=w1162, spreadsheet string=w1160, array type (2D Dbl)=w1158) -> (array=w1159:string[])  [unwired: 1 in]
        n337 = call "4155C Write array to file.vi"("Byte Stream File Refnum"=w1167, "Header"=w1159, "Data Array"=w1182, "error in (no error)"=w1168) -> ("dup refnum"=w1165:refnum<file>, "error out"=w1166:errorcluster)  [unwired: 1 in]
        n338 = Close File(refnum=w1165, error in=w1166) -> (error out=w1154:errorcluster)  [unwired: 1 out]
      }
      frame "serial" {
        n339 = local read "Termination char\n(0xA = '\\n' = LF)\n(0xD = '\\r' = CR)"() -> (w1214:u8)
        n340 = Index Array(array=w1221, index=0 ("Index")) -> (element=w1220:string)
        n341 = local read "Enable Termination\nChar (T)"() -> (w1215:bool)
        n342 = local read "parity"() -> (w1207:u16)
        n343 = local read "Delay before read (ms)"() -> (w1213:u32)
        n344 = local read "byte count"() -> (w1211:u32)
        n345 = local read "Timeout (ms)"() -> (w1212:u32)
        n346 = local read "VISA resource name"() -> (w1209:refnum<visa-resource-name>)
        n347 = local read "baud rate"() -> (w1208:u32)
        n348 = local read "Serial End Mode for Reads"() -> (w1206:u16)
        n349 = local read "data bits"() -> (w1205:u16)
        n350 = local read "stop bits"() -> (w1204:u16)
        n351 = local read "flow control"() -> (w1210:u16)
        n352 = call "Serial write and read v0.5.vi"("Delay before read (ms)"=w1213, "Termination char\n(0xA = '\\n' = LF)\n(0xD = '\\r' = CR)"=w1214, "Enable Termination\nChar (T)"=w1215, "parity"=w1207, "stop bits"=w1204, "string to write"=w1220, "flow control"=w1210, "byte count"=w1211, "Serial Settings:Serial End Mode for Reads"=w1206, "Timeout (ms)"=w1212, "error in (no error)"=w1226, "VISA resource name"=w1209, "baud rate"=w1208, "data bits"=w1205) -> ("Serial port output"=w1218:string, "error out"=w1225:errorcluster)
        n353 = Build Array (concatenate)(w1218, w1216) -> (w1217:string[])
      }
    }
    n354 = Build Array("Time /s" ("element"), "Id max /A" ("VAR2 Name"), "Id min /A" ("VAR2 Name")) -> (w86:string[])
    n355 = Build Array(w81, w80, w74) -> (w79:dbl[][])
    n356 = Concatenate Strings(w52, "-Serial port output", ".txt" ("Suffix")) -> (w56:string)
    n357 = Array To Spreadsheet String(array=w57, 3:"" ("format string")) -> (spreadsheet string=w62:string)  [unwired: 1 in]
    n358 = Transpose 2D Array(2D array=w79) -> (transposed array=w78:dbl[][])
    n359 = String To Path(string=w56) -> (path=w53:path)
    n360 = Concatenate Strings(w52, "-Ion-Ioff", ".txt" ("Suffix")) -> (w94:string)
    n361 = Array To Spreadsheet String(array=w86, 3:"" ("format string")) -> (spreadsheet string=w85:string)  [unwired: 1 in]
    n362 = Array To Spreadsheet String(array=w78, 3:"%e" ("format string")) -> (spreadsheet string=w84:string)  [unwired: 1 in]
    n363 = String To Path(string=w94) -> (path=w93:path)
    n364 = local write "Serial port output"(w62) -> ()
    n365 = Write to Text File(file (use dialog)=w53, text=w57, error in=w51) -> (refnum out=w58:refnum<file>, error out=w59:errorcluster)  [unwired: 1 in, 1 out]
    n366 = Build Array(w85, w84) -> (w83:string[])
    n367 = Close File(refnum=w58, error in=w59) -> (error out=w50:errorcluster)  [unwired: 1 out]
    n368 = Write to Text File(file (use dialog)=w93, text=w83, error in=w50) -> (refnum out=w95:refnum<file>, error out=w82:errorcluster)  [unwired: 1 in, 1 out]
    n369 = Close File(refnum=w95, error in=w82) -> (error out=w76:errorcluster)  [unwired: 1 out]
  }
  "error out" <- w9
